vi "FPGA Target_PCIe_7856R.vi"() -> ()   [LabVIEW 2023]
uses:
  <vilib>/Platform/TimedLoop/XDataNode/timing_clust.ctl
  <vilib>/Platform/TimedLoop/XDataNode/nitl_modes.ctl
  <vilib>/Platform/TimedLoop/XDataNode/wakeup.ctl
  <vilib>/rvi/Emulation/niFpgaSctlEmulationGetInTimedLoop.vi
  <vilib>/rvi/Emulation/niFpgaProcessEmulError.vi
  <vilib>/rvi/eio/common/nirviEmuTemplateMethod_errors.vi
  <vilib>/rvi/Emulation/niFpgaGetClockAttributes.vi
  <vilib>/rvi/Emulation/niFpgaEmulationReportErrorSimple.vi
  <vilib>/eio/utilities/niEioResolveVilibRelativePath.vi
  <vilib>/rvi/interface/RandomDataEmulation/niFpgaRandomDataHandleErrors.vi
  <vilib>/rvi/Emulation/niFpgaCriticalErrorInLSC.vi
  Tick Count.vi
  <vilib>/rvi/Memory/Memory_Emulation/nirvimemoryFastEmulation.vi
  <vilib>/rvi/Memory/Memory_Emulation/nirvimemoryEmulation.vi
  <vilib>/rvi/Emulation/niFpgaEmulationIsFPGAContextNoSignature.vi
  <vilib>/rvi/DataTransferAndStorage/Container/Common/niFpgaContainerGetUniqueNameForEmu.vi
  <vilib>/rvi/errors/nirviReportUnexpectedCaseInternalError (U32).vi
  <vilib>/eio/EIONode/EIONode.xnode
  <vilib>/rvi/DataTransferAndStorage/Container/XNode/niFpgaContainer.xnode
  <vilib>/rvi/interface/RandomDataEmulation/nirviRandomDataFpgaReadWriteTemplate.vi
  <vilib>/Platform/TimedLoop/XDataNode/XDataNode.xnode
  <vilib>/rvi/Arithmetic/AddSubMult/XNode/nirviSatArithmetic.xnode
  <vilib>/Platform/TimedLoop/XDataNode/XDNodeRunTimeDep.lvlib
panel:
  out "Move Z Picomotor Direction":bool
  out "Move Z Picomotor":bool
  out "Tick Count(Ticks)":u32
  in  "HoldTimerScale":u64=18446744073709526080
  in  "Feedback1 on  Hold":bool
  out "Feedback2 Error":i32
  out "Feedback1 Error":i32
  out "Feedback2 Boolean":bool
  out "Feedback1 Boolean":bool
  out "ExtraTime 4":fxp<+,64,64>
  in  "DistanceToBulk 3":i16
  in  "DistanceToBulk 2":i16
  out "HasHeldHoldTimeHappend?":bool
  out "Z_axis_-10Vto10V":bool
  out "TraceRetraceFirstUse":bool
  in  "DistanceToBulk":i16
  out "V START":i16
  out "V END":i16
  out "X START":i16
  out "Y START":i16
  out "Z START":i16
  out "X END":i16
  out "Y END":i16
  out "Z END":i16
  out "V2 START":i16
  out "Count Average":i16
  out "AverageSum":i64
  out "IterateHolder":i16
  out "V2 VEl":i16
  out "V2 END":i16
  out "Update Position Loop Wait Time (ms)":u16=1
  out "LineType":i16
  out "V VEl":i16
  out "Z VEL":i16
  out "Y VEL":i16
  out "X VEL":i16
  out "Element":i16
  in  "V on Fly":i16=-32768
  in  "Change V on Fly":bool
  in  "Feedback_Threshold":i64
  in  "FeedBackType":u8
  out "x < y?":bool
  out "ExtraTime 3":fxp<+,64,64>
  in  "P2AvgMinus":i32
  out "ExtraTime 2":fxp<+,64,64>
  in  "P2AvgWhole":i32
  in  "Xoffset":u32
  in  "P":fxp<+/-,32,1>
  in  "Upper limit Of dZ":i32
  in  "FeedBackType 2":u8
  in  "Feedback_Threshold 2":i32
  in  "GreaterThan 2":bool
  in  "GreaterThan":bool
  in  "V2 on Fly":i16=-32768
  in  "Change V on Fly 2":bool
  out "CurrentMeasuredX":i16
  in  "2^(-n)":i16
  out "SampleNum":i16
  in  "Buffer Loop Wait Time (tICKS)":u32=1
  out "SampleIterator":i16
  out "Internal Stop":bool caption="Stop"
  out "MeasuredCurrent":i16=32767
  out "Applied Voltage":i16=-32768
  in  "External Stop":bool caption="Stop"
  in  "External Pause":bool
  out "Applied Z":i16
  out "Applied Y":i16
  out "Applied X":i16
  in  "Internal Pause":bool
  out "Accum Z":i32
  out "Accum I":i32
  out "Accum dV":i32
  out "Accum I2":i32
  out "OnlyStopLineONCE X":bool
  out "Accum Ext ac":i32
  out "Ext amp":i16=32767
  out "Accum Ext phase":i32
  in  "ExpandVelScaller X":i16=-27
  out "LineNumber":u64
  out "WaitingForWayPoints":bool caption="Stop"
  out "HoldTimer (ticks)":u64
  out "MeasuredCurrent 2":i16=32767
  out "Ext Phase":i16=32767
  in  "ExpandVelScaller Y":i16=-27
  in  "ExpandVelScaller Z":i16=-27
  in  "ExpandVelScaller V":i16=-27
  out "Accum I3":i32
  out "MeasuredCurrent 3":i16=32767
  out "MeasuredCurrent 4":i16=32767
  out "Accum Y":i32
  out "Accum X":i32
  out "OnlyStopLineONCE Y":bool
  out "OnlyStopLineONCE Z":bool
  out "OnlyStopLineONCE V":bool
  in  "EndCurrentLine":bool
  out "StopMoveX":bool
  out "StopMoveY":bool
  out "StopMoveZ":bool
  out "StopMoveV":bool
  out "Jump V":bool
  out "Stop Hold Position":bool
  out "Applied Voltage 2":i16
  out "StopMoveV2":bool
  out "Accum dV2":i32
  out "Jump V2":bool
  in  "ExpandVelScaller V2":i16=-27
  out "OnlyStopLineONCE V2":bool
  out "MoveAverage":i16
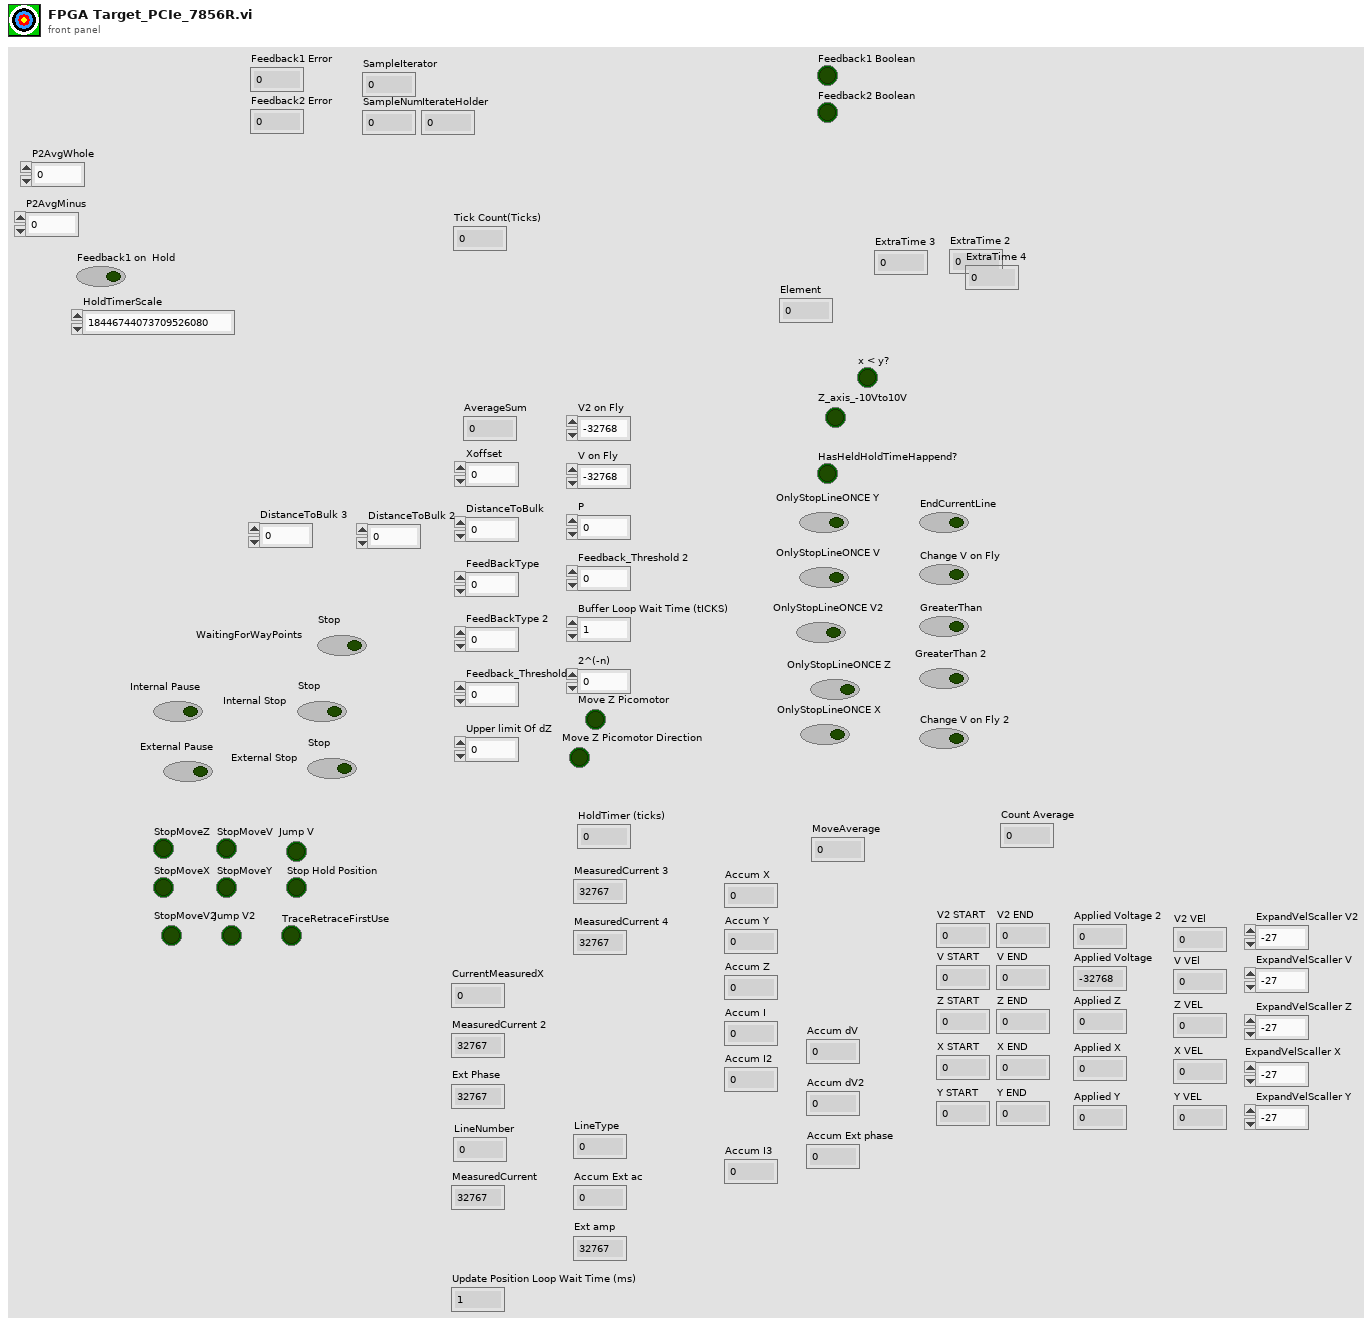
[diagram p1: front panel]
types:
  T1 = typedef "XDNodeRunTimeDep.lvlib/timing_clust.ctl" = cluster{"Expected End [f-1]":u64, "Actual End [f-1]":u64, "Finished Late? [f-1]":bool, "Expected End [i-1]":u64, "Actual End [i-1]":u64, "Finished Late? [i-1]":bool, "Expected Start [i]":u64, "Actual Start [i]":u64, "Expected Start [f]":u64, "Actual Start [f]":u64, "Source Name":string, "Structure Name":string, "Period":i64, "Deadline":i64, "Offset":i64, "Start":i64, "Priority":i32, "Timeout":i32, "Mode":T2, "Wakeup Reason":T3, "Error":errorcluster, "Source Type":string, "Secondary Source Type":string, "Global End Time":u64, "Global Start Time":u64, "Frame Duration":u64, "Iteration Duration":u64, "Assigned CPU":i32, "I/O Scan Engine Mode":u32}
  T2 = typedef "XDNodeRunTimeDep.lvlib/nitl_modes.ctl" = enum32{"No Change", "Process missed periods, maintain original phase", "Discard missed periods, maintain original phase", "Process missed periods, ignore original phase", "Discard missed periods, ignore original phase"}
  T3 = typedef "XDNodeRunTimeDep.lvlib/wakeup.ctl" = enum32{"Normal", "Aborted", "Asynchronous wakeup", "Timing source error", "Timed loop error", "Timeout"}
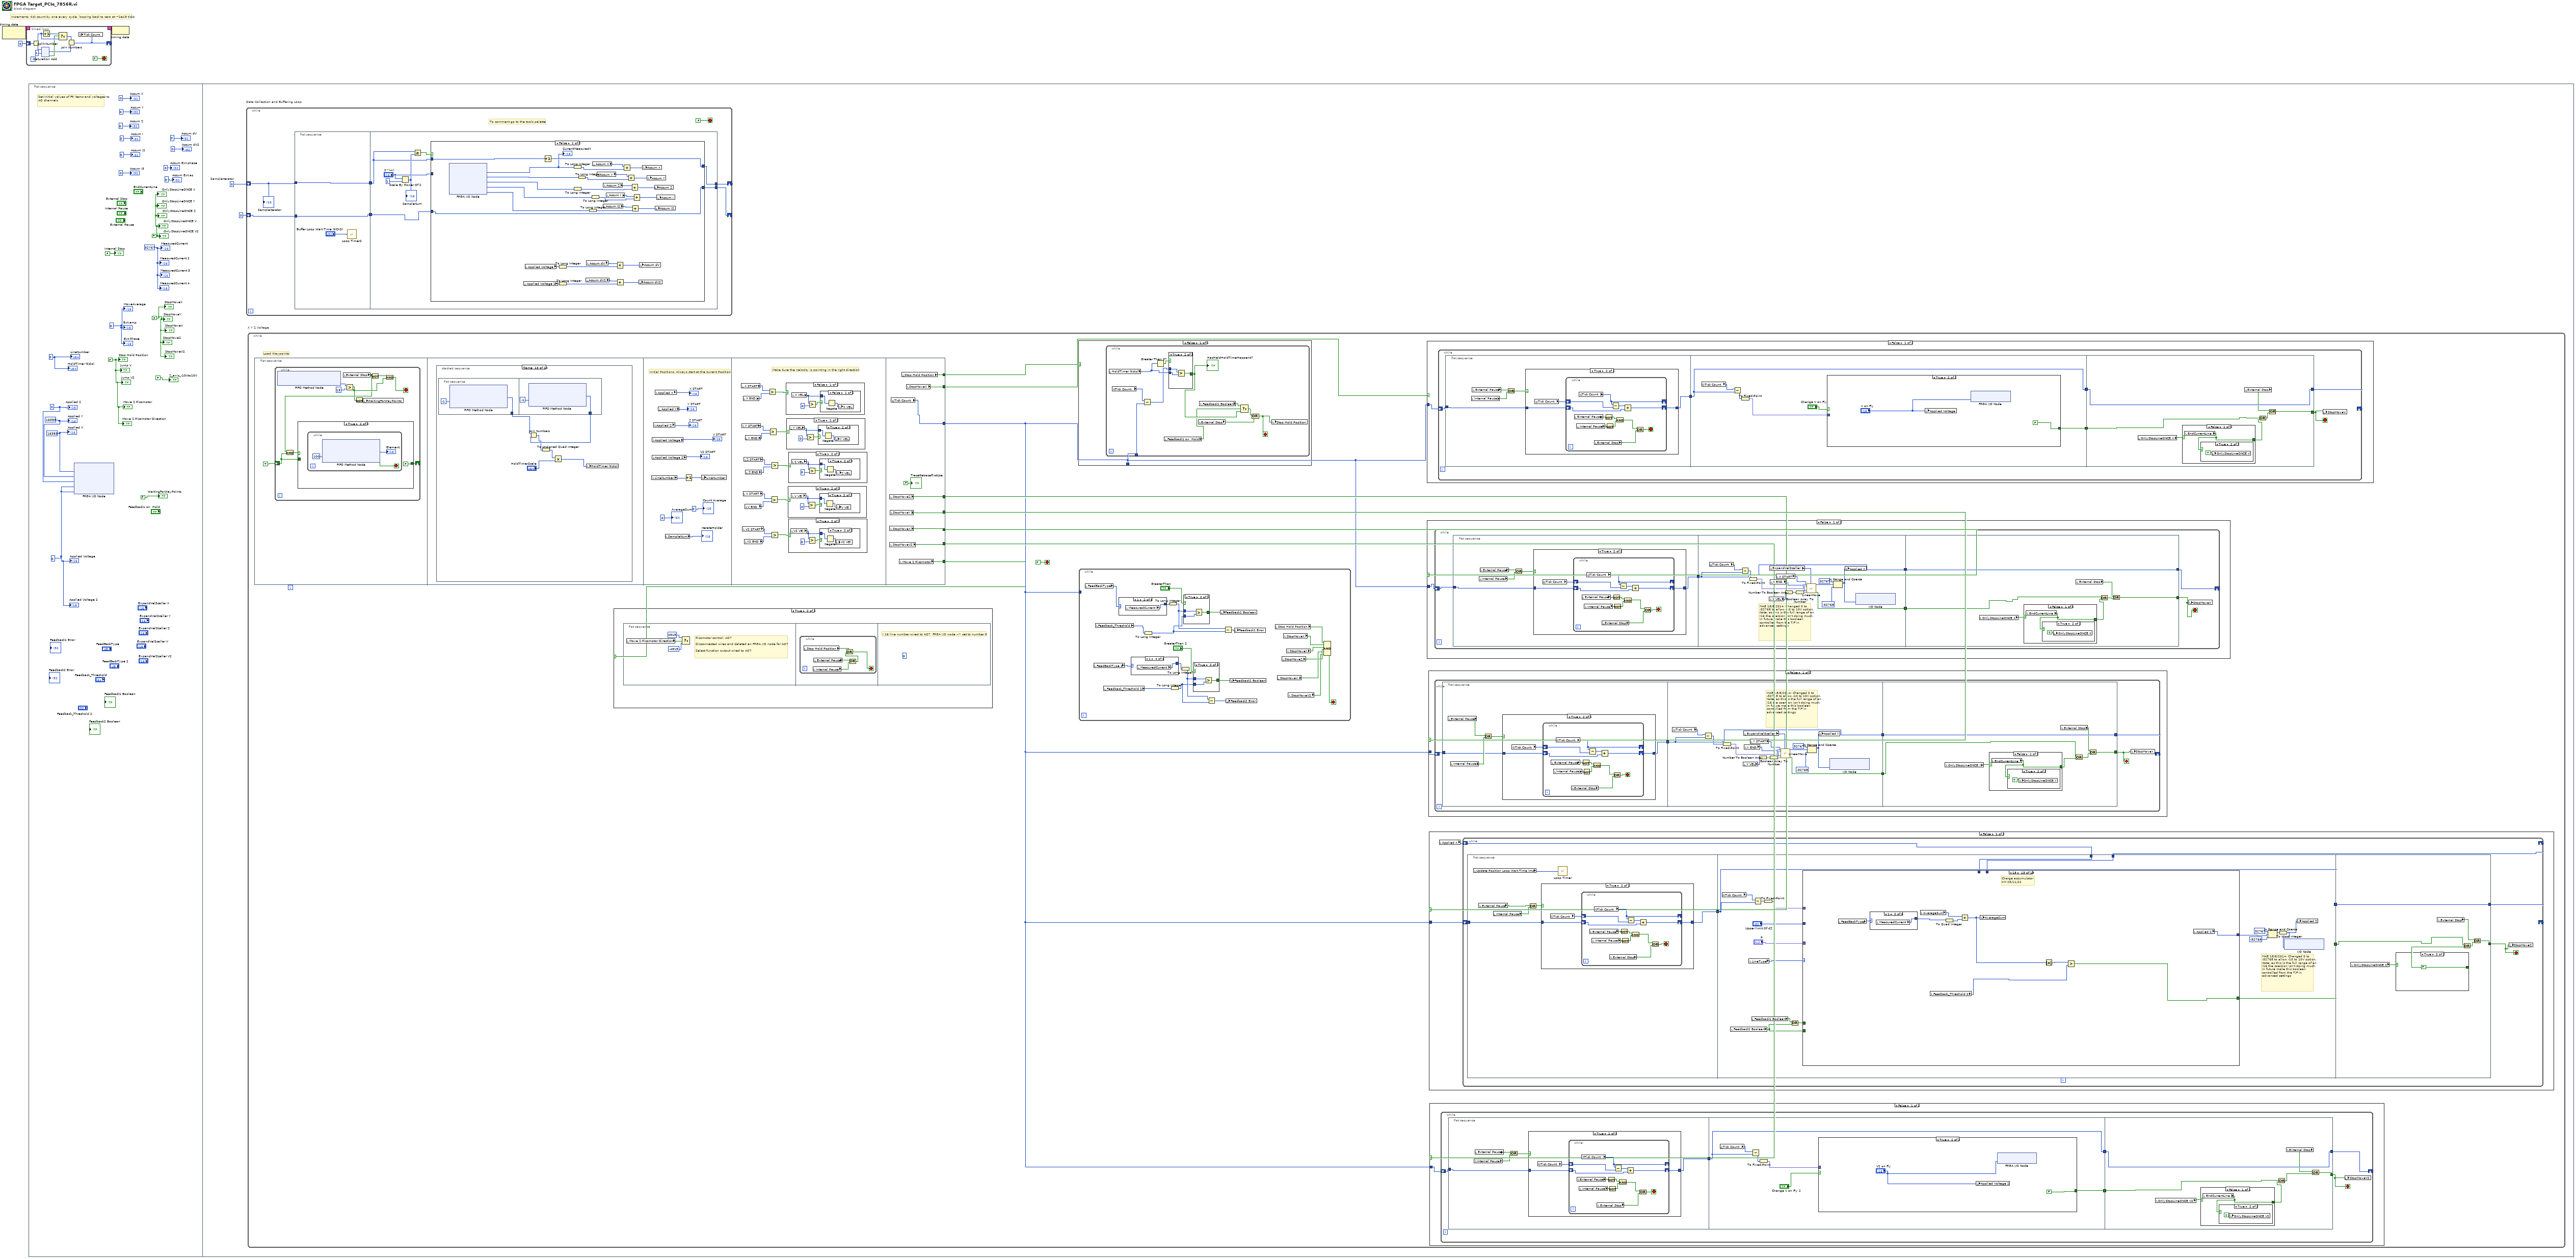
[diagram p0: block diagram]
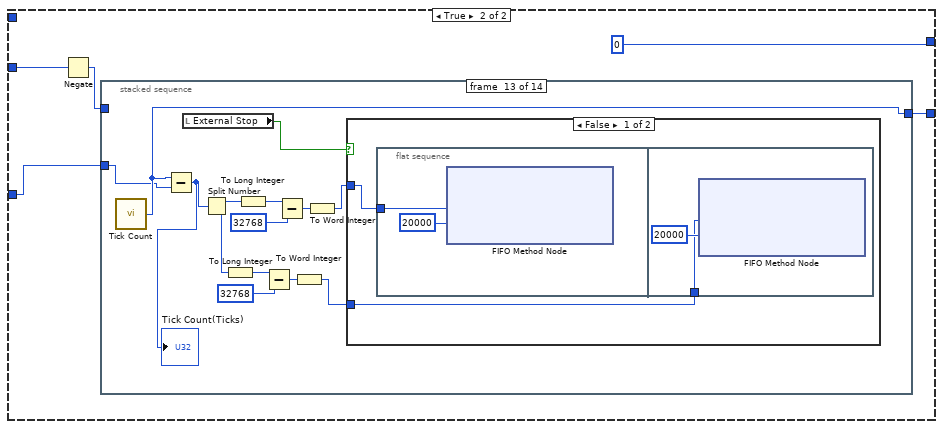
[diagram p2: hidden frame]
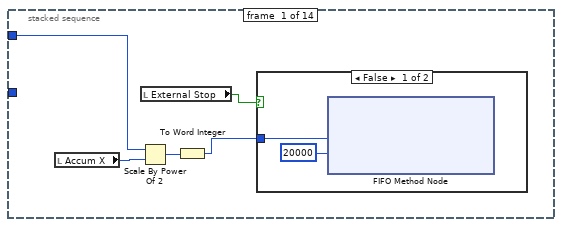
[diagram p3: hidden frame]
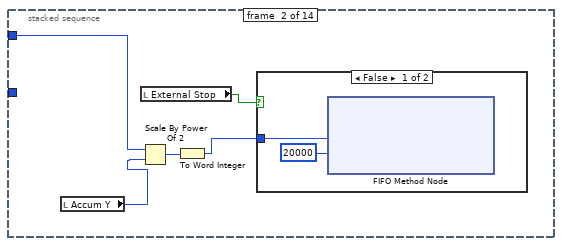
[diagram p5: hidden frame]
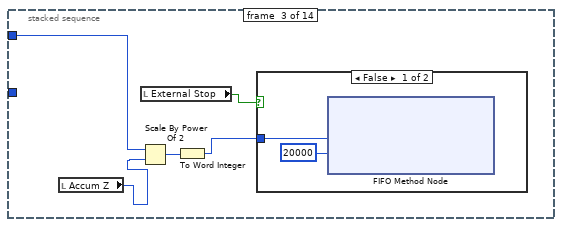
[diagram p7: hidden frame]
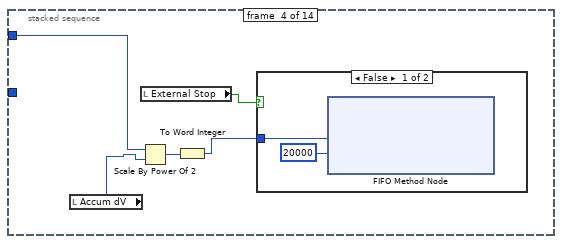
[diagram p9: hidden frame]
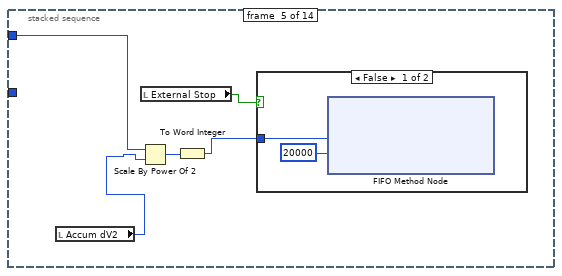
[diagram p11: hidden frame]
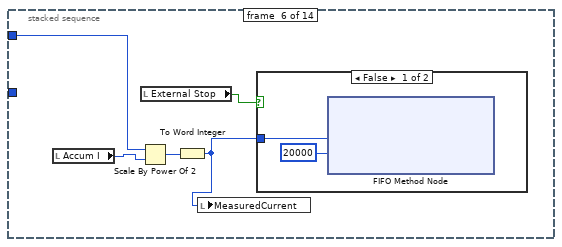
[diagram p13: hidden frame]
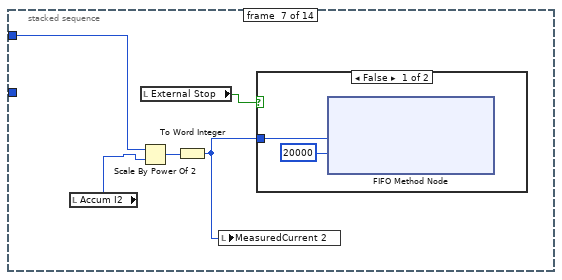
[diagram p15: hidden frame]
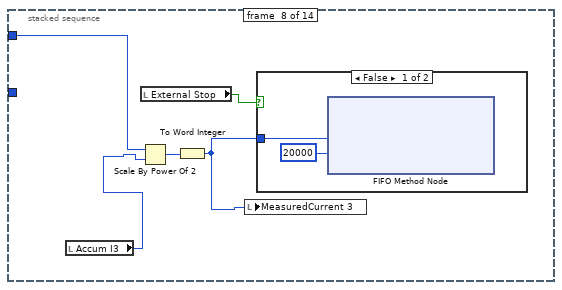
[diagram p17: hidden frame]
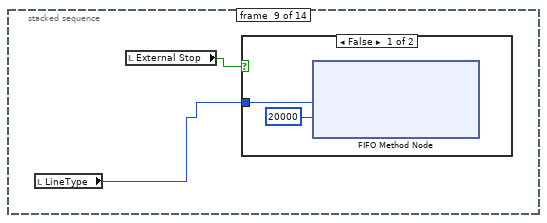
[diagram p19: hidden frame]
diagram:
  # "Increments  tick count by one every cycle, looping back to zero at ~2e19 ticks"
  n1 = node-c288() -> (w3:T1)  [unwired: 1 in]
  n2 = timed-loop {
    timing: w3 -> [_]
    timing-out: [_] -> w2
    shift-right: [w5] -> _
    shift-left: u64 0 -> [w13]
    stop <- FALSE stop-if-true
    n3 = Split Number(x=w13) -> (hi(x)=w10:u32, lo(x)=w12:u32)
    n4 = xnode "Saturation Add"("x"=w12, "y"=u32 1) -> ("x+y"=w6:u32, "overflow"=w7:bool)
    n5 = Increment(x=w10) -> (x+1=w11:u32)
    n6 = Select(t=w11, s=w7, f=w10) -> (s? t:f=w9:u32)
    n7 = Join Numbers(hi=w9, lo=w6) -> ((hi.lo)=w5:u64)
    n8 = global write "Tick Count.vi" "Tick Count"(w5) -> ()
  }
  n9 = flat-sequence {
    frame #0 {
      w28 = i16 0 ("Applied Voltage")
      w33 = FALSE ("OnlyStopLineONCE V2")
      w34 = FALSE ("Internal Stop")
      w29 = FALSE ("Internal Stop")
      w36 = i16 0 ("Applied Volatge")
      w37 = i16 16383 ("Applied Volatge")
      w38 = i16 16383 ("Applied Volatge")
      w32 = u64 0 ("LineNumber")
      w31 = i16 0 ("Ext amp")
      w41 = i16 32767 ("dZ Position")
      # "Set initial values of FP items and voltages to AO channels"
      n10 = xnode "FPGA I/O Node"("Connector0/AO0"=w38, "Connector0/AO1"=w37, "Connector0/AO2"=w36, "Connector0/AO3"=w28, "Connector0/AO4"=w28) -> ()  [unwired: 5 in, 5 out]
      "Internal Stop" <- FALSE ("Internal Stop")
      "MeasuredCurrent" <- w41
      "Applied Voltage" <- w28
      "Applied Z" <- w36
      "Applied Y" <- w37
      "Applied X" <- w38
      "Accum Z" <- 0 ("Applied Volatge")
      "Accum I" <- 0 ("Applied Volatge")
      "Accum dV" <- 0 ("Applied Volatge")
      "Accum I2" <- 0 ("Applied Volatge")
      "OnlyStopLineONCE X" <- w33
      "Accum Ext ac" <- 0 ("Accum Ext ac")
      "Ext amp" <- w31
      "Accum Ext phase" <- 0 ("Accum Ext phase")
      "LineNumber" <- w32
      "WaitingForWayPoints" <- FALSE ("WaitingForWayPoints")
      "HoldTimer (ticks)" <- w32
      "MeasuredCurrent 2" <- w41
      "Ext Phase" <- w31
      "Accum I3" <- 0 ("Applied Volatge")
      "MeasuredCurrent 3" <- w41
      "MeasuredCurrent 4" <- w41
      "Accum Y" <- 0 ("Applied Volatge")
      "Accum X" <- 0 ("Applied Volatge")
      "OnlyStopLineONCE Y" <- w33
      "OnlyStopLineONCE Z" <- w33
      "OnlyStopLineONCE V" <- w33
      "StopMoveX" <- w34
      "StopMoveY" <- w34
      "StopMoveZ" <- w34
      "StopMoveV" <- w34
      "Jump V" <- w29
      "Stop Hold Position" <- w29
      "Applied Voltage 2" <- w28
      "StopMoveV2" <- w34
      "Accum dV2" <- 0 ("Applied Volatge")
      "Jump V2" <- w29
      "OnlyStopLineONCE V2" <- w33
      "MoveAverage" <- w31
      "Z_axis_-10Vto10V" <- FALSE ("Internal Stop")
      "Move Z Picomotor" <- w29
      "Move Z Picomotor Direction" <- w29
    }
    frame #1 {
      w52 = i16 0  # SampleIterator
      n11 = while "Data Collection and Buffering Loop" {
        shift-right: [w57] -> _
        shift-left: w52 -> [w58]
        shift-right: [w55] -> _
        shift-left: u32 0 ("Tick Count(Ticks)") -> [w53]
        stop <- FALSE stop-if-true
        # "To comment go to the tools palette"
        n12 = flat-sequence {
          tunnel: [w62] -> w59
          tunnel: w58 -> [w62]
          tunnel: w53 -> [w60]
          tunnel: [w60] -> w54
          tunnel: w59 -> [w70]
          tunnel: [w69] -> w57
          tunnel: [w64] -> w55
          tunnel: w54 -> [w63]
          frame #0 {
            n13 = call "Loop Timer2"("Count(Ticks)"="Buffer Loop Wait Time (tICKS)") -> ()  [unwired: 1 out]
          }
          frame #1 {
            n14 = Scale By Power Of 2(n="2^(-n)", x=i16 1) -> (x*2^n=w67:i16)
            "SampleNum" <- w67
            n15 = Greater Or Equal?(x=w70, y=w67) -> (x >= y?=w65:bool)
            n16 = case shown="False" w65 {
              tunnel: w70 -> [w101 _]
              tunnel: [w100 i16 0 ("lo")] -> w69
              tunnel: "2^(-n)" -> [_ w105]
              tunnel: [w73 w103] -> w64
              tunnel: w63 -> [w73 w102]
              frame False {
                n17 = xnode "FPGA I/O Node"() -> ("Connector0/AI0"=w78:i16, "Connector0/AI1"=w85:i16, "Connector0/AI2"=w88:i16, "Connector0/AI3"=w72:i16, "Connector0/AI4"=w71:i16)  [unwired: 5 in, 5 out]
                "CurrentMeasuredX" <- w78
                n18 = local read "Applied Voltage 2"() -> (w76:i16)
                n19 = local read "Applied Voltage"() -> (w90:i16)
                n20 = Increment(x=w101) -> (x+1=w100:i16)
                n21 = To Long Integer(number=w90) -> (32bit integer=w89:i32)
                n22 = To Long Integer(number=w76) -> (32bit integer=w77:i32)
                n23 = To Long Integer(number=w88) -> (32bit integer=w86:i32)
                n24 = To Long Integer(number=w78) -> (32bit integer=w79:i32)
                n25 = To Long Integer(number=w85) -> (32bit integer=w84:i32)
                n26 = local read "Accum dV2"() -> (w74:i32)
                n27 = local read "Accum dV"() -> (w92:i32)
                n28 = To Long Integer(number=w71) -> (32bit integer=w94:i32)
                n29 = To Long Integer(number=w72) -> (32bit integer=w97:i32)
                n30 = local read "Accum X"() -> (w80:i32)
                n31 = local read "Accum Y"() -> (w83:i32)
                n32 = local read "Accum I2"() -> (w95:i32)
                n33 = local read "Accum Z"() -> (w87:i32)
                n34 = local read "Accum I"() -> (w98:i32)
                n35 = Add(x=w92, y=w89) -> (x+y=w91:i32)
                n36 = Add(x=w74, y=w77) -> (x+y=w75:i32)
                n37 = Add(x=w80, y=w79) -> (x+y=w81:i32)
                n38 = Add(x=w83, y=w84) -> (x+y=w82:i32)
                n39 = Add(x=w87, y=w86) -> (x+y=w99:i32)
                n40 = Add(x=w95, y=w94) -> (x+y=w93:i32)
                n41 = Add(x=w98, y=w97) -> (x+y=w96:i32)
                n42 = local write "Accum dV2"(w75) -> ()
                n43 = local write "Accum dV"(w91) -> ()
                n44 = local write "Accum X"(w81) -> ()
                n45 = local write "Accum Y"(w82) -> ()
                n46 = local write "Accum Z"(w99) -> ()
                n47 = local write "Accum I2"(w93) -> ()
                n48 = local write "Accum I"(w96) -> ()
              }
              frame True {
                n49 = Negate(x=w105) -> (-x=w104:i16)
                n50 = stacked-sequence {
                  tunnel: w104 -> [w107 w115 w122 w130 w137 w144 w151 w158 _ _ w175 w182 _ _]
                  tunnel: [_ _ _ _ _ _ _ _ _ _ _ _ w188 _] -> w103
                  tunnel: w102 -> [_ _ _ _ _ _ _ _ _ _ _ _ w187 _]
                  frame #0 {
                    n51 = local read "Accum X"() -> (w108:i32)
                    n52 = Scale By Power Of 2(n=w107, x=w108) -> (x*2^n=w109:i32)
                    n53 = local read "External Stop"() -> (w110:bool)
                    n54 = To Word Integer(number=w109) -> (16bit integer=w111:i16)
                    n55 = case shown="False" w110 {
                      tunnel: w111 -> [w112 _]
                      frame False {
                        n56 = xnode ("FIFO Method Node")("Element"=w112, "Timeout"=20000) -> ()  [unwired: 1 in, 2 out]
                      }
                      frame True {
                      }
                    }
                  }
                  frame #1 {
                    n57 = local read "Accum Y"() -> (w114:i32)
                    n58 = Scale By Power Of 2(n=w115, x=w114) -> (x*2^n=w116:i32)
                    n59 = local read "External Stop"() -> (w117:bool)
                    n60 = To Word Integer(number=w116) -> (16bit integer=w118:i16)
                    n61 = case shown="False" w117 {
                      tunnel: w118 -> [w119 _]
                      frame False {
                        n62 = xnode ("FIFO Method Node")("Element"=w119, "Timeout"=20000) -> ()  [unwired: 1 in, 2 out]
                      }
                      frame True {
                      }
                    }
                  }
                  frame #2 {
                    n63 = local read "Accum Z"() -> (w121:i32)
                    n64 = Scale By Power Of 2(n=w122, x=w121) -> (x*2^n=w123:i32)
                    n65 = local read "External Stop"() -> (w124:bool)
                    n66 = To Word Integer(number=w123) -> (16bit integer=w125:i16)
                    n67 = case shown="False" w124 {
                      tunnel: w125 -> [w126 _]
                      frame False {
                        n68 = xnode ("FIFO Method Node")("Element"=w126, "Timeout"=20000) -> ()  [unwired: 1 in, 2 out]
                      }
                      frame True {
                      }
                    }
                  }
                  frame #3 {
                    n69 = local read "Accum dV"() -> (w128:i32)
                    n70 = Scale By Power Of 2(n=w130, x=w128) -> (x*2^n=w131:i32)
                    n71 = local read "External Stop"() -> (w132:bool)
                    n72 = To Word Integer(number=w131) -> (16bit integer=w129:i16)
                    n73 = case shown="False" w132 {
                      tunnel: w129 -> [w133 _]
                      frame False {
                        n74 = xnode ("FIFO Method Node")("Element"=w133, "Timeout"=20000) -> ()  [unwired: 1 in, 2 out]
                      }
                      frame True {
                      }
                    }
                  }
                  frame #4 {
                    n75 = local read "Accum dV2"() -> (w135:i32)
                    n76 = Scale By Power Of 2(n=w137, x=w135) -> (x*2^n=w138:i32)
                    n77 = local read "External Stop"() -> (w139:bool)
                    n78 = To Word Integer(number=w138) -> (16bit integer=w136:i16)
                    n79 = case shown="False" w139 {
                      tunnel: w136 -> [w140 _]
                      frame False {
                        n80 = xnode ("FIFO Method Node")("Element"=w140, "Timeout"=20000) -> ()  [unwired: 1 in, 2 out]
                      }
                      frame True {
                      }
                    }
                  }
                  frame #5 {
                    n81 = local read "Accum I"() -> (w143:i32)
                    n82 = Scale By Power Of 2(n=w144, x=w143) -> (x*2^n=w145:i32)
                    n83 = local read "External Stop"() -> (w146:bool)
                    n84 = To Word Integer(number=w145) -> (16bit integer=w142:i16)
                    n85 = local write "MeasuredCurrent"(w142) -> ()
                    n86 = case shown="False" w146 {
                      tunnel: w142 -> [w147 _]
                      frame False {
                        n87 = xnode ("FIFO Method Node")("Element"=w147, "Timeout"=20000) -> ()  [unwired: 1 in, 2 out]
                      }
                      frame True {
                      }
                    }
                  }
                  frame #6 {
                    n88 = local read "Accum I2"() -> (w150:i32)
                    n89 = Scale By Power Of 2(n=w151, x=w150) -> (x*2^n=w152:i32)
                    n90 = local read "External Stop"() -> (w153:bool)
                    n91 = To Word Integer(number=w152) -> (16bit integer=w149:i16)
                    n92 = local write "MeasuredCurrent 2"(w149) -> ()
                    n93 = case shown="False" w153 {
                      tunnel: w149 -> [w154 _]
                      frame False {
                        n94 = xnode ("FIFO Method Node")("Element"=w154, "Timeout"=20000) -> ()  [unwired: 1 in, 2 out]
                      }
                      frame True {
                      }
                    }
                  }
                  frame #7 {
                    n95 = local read "Accum I3"() -> (w157:i32)
                    n96 = Scale By Power Of 2(n=w158, x=w157) -> (x*2^n=w159:i32)
                    n97 = local read "External Stop"() -> (w160:bool)
                    n98 = To Word Integer(number=w159) -> (16bit integer=w156:i16)
                    n99 = local write "MeasuredCurrent 3"(w156) -> ()
                    n100 = case shown="False" w160 {
                      tunnel: w156 -> [w161 _]
                      frame False {
                        n101 = xnode ("FIFO Method Node")("Element"=w161, "Timeout"=20000) -> ()  [unwired: 1 in, 2 out]
                      }
                      frame True {
                      }
                    }
                  }
                  frame #8 {
                    n102 = local read "LineType"() -> (w163:i16)
                    n103 = local read "External Stop"() -> (w164:bool)
                    n104 = case shown="False" w164 {
                      tunnel: w163 -> [w165 _]
                      frame False {
                        n105 = xnode ("FIFO Method Node")("Element"=w165, "Timeout"=20000) -> ()  [unwired: 1 in, 2 out]
                      }
                      frame True {
                      }
                    }
                  }
                  frame #9 {
                    n106 = local read "LineNumber"() -> (w168:u64)
                    n107 = local read "External Stop"() -> (w169:bool)
                    n108 = To Word Integer(number=w168) -> (16bit integer=w167:i16)
                    n109 = case shown="False" w169 {
                      tunnel: w167 -> [w170 _]
                      frame False {
                        n110 = xnode ("FIFO Method Node")("Element"=w170, "Timeout"=20000) -> ()  [unwired: 1 in, 2 out]
                      }
                      frame True {
                      }
                    }
                  }
                  frame #10 {
                    n111 = local read "Accum Ext ac"() -> (w174:i32)
                    n112 = local read "External Stop"() -> (w176:bool)
                    n113 = Scale By Power Of 2(n=w175, x=w174) -> (x*2^n=w173:i32)
                    n114 = To Word Integer(number=w173) -> (16bit integer=w172:i16)
                    n115 = case shown="False" w176 {
                      tunnel: w172 -> [w177 _]
                      frame False {
                        n116 = xnode ("FIFO Method Node")("Element"=w177, "Timeout"=20000) -> ()  [unwired: 1 in, 2 out]
                      }
                      frame True {
                      }
                    }
                    n117 = local write "Ext amp"(w172) -> ()
                  }
                  frame #11 {
                    n118 = local read "Accum Ext phase"() -> (w180:i32)
                    n119 = local read "External Stop"() -> (w183:bool)
                    n120 = Scale By Power Of 2(n=w182, x=w180) -> (x*2^n=w181:i32)
                    n121 = To Word Integer(number=w181) -> (16bit integer=w179:i16)
                    n122 = local write "Ext Phase"(w179) -> ()
                    n123 = case shown="False" w183 {
                      tunnel: w179 -> [w184 _]
                      frame False {
                        n124 = xnode ("FIFO Method Node")("Element"=w184, "Timeout"=20000) -> ()  [unwired: 1 in, 2 out]
                      }
                      frame True {
                      }
                    }
                  }
                  frame #12 {
                    n125 = call "Tick Count"() -> ("Tick Count(Ticks)"=w188:u32)
                    n126 = Subtract(x=w188, y=w187) -> (x-y=w186:u32)
                    "Tick Count(Ticks)" <- w186
                    n127 = local read "External Stop"() -> (w199:bool)
                    n128 = Split Number(x=w186) -> (hi(x)=w198:u16, lo(x)=w190:u16)
                    n129 = To Long Integer(number=w190) -> (32bit integer=w191:i32)
                    n130 = To Long Integer(number=w198) -> (32bit integer=w197:i32)
                    n131 = Subtract(x=w191, y=32768) -> (x-y=w193:i32)
                    n132 = Subtract(x=w197, y=32768) -> (x-y=w195:i32)
                    n133 = To Word Integer(number=w193) -> (16bit integer=w189:i16)
                    n134 = To Word Integer(number=w195) -> (16bit integer=w194:i16)
                    n135 = case shown="False" w199 {
                      tunnel: w194 -> [w201 _]
                      tunnel: w189 -> [w200 _]
                      frame False {
                        n136 = flat-sequence {
                          tunnel: w201 -> [w202]
                          tunnel: w200 -> [w204]
                          frame #0 {
                            n137 = xnode ("FIFO Method Node")("Element"=w202, "Timeout"=20000) -> ()  [unwired: 1 in, 2 out]
                          }
                          frame #1 {
                            n138 = xnode ("FIFO Method Node")("Element"=w204, "Timeout"=20000) -> ()  [unwired: 1 in, 2 out]
                          }
                        }
                      }
                      frame True {
                      }
                    }
                  }
                  frame #13 {
                    n139 = local write "Accum dV"(0 ("MeasuredCurrent")) -> ()
                    n140 = local write "Accum Z"(0 ("MeasuredCurrent")) -> ()
                    n141 = local write "Accum dV2"(0 ("Accum Ext ac")) -> ()
                    n142 = local write "Accum I2"(0 ("MeasuredCurrent")) -> ()
                    n143 = local write "Accum I"(0 ("MeasuredCurrent")) -> ()
                    n144 = local write "Accum Y"(0 ("Accum Ext ac")) -> ()
                    n145 = local write "Accum X"(0 ("MeasuredCurrent")) -> ()
                    n146 = local write "Accum Ext ac"(0 ("Accum Ext ac")) -> ()
                    n147 = local write "Accum I3"(0 ("Accum Ext ac")) -> ()
                    n148 = local write "Accum Ext phase"(0 ("Accum Ext phase")) -> ()
                  }
                }
              }
            }
          }
        }
        "SampleIterator" <- w58
      }
      n149 = while "X Y Z Voltage" {
        stop <- FALSE stop-if-true
        # "Load Waypoints"
        n150 = flat-sequence {
          tunnel: [w1142] -> w217
          tunnel: [w1141] -> w223
          tunnel: [w1140] -> w222
          tunnel: [w1139] -> w221
          tunnel: [w1138] -> w220
          tunnel: [w1137] -> w219
          tunnel: [w1135] -> w218
          tunnel: [w1134] -> w216
          frame #0 {
            n151 = while {
              shift-right: [w938] -> _
              shift-left: TRUE ("WaitingForWayPoints") -> [w939]
              stop <- w942 stop-if-true
              n152 = xnode ("FIFO Method Node")() -> ("Number of Elements to Read"=w947:u32)  [unwired: 1 in, 1 out]
              n153 = local read "External Stop"() -> (w940:bool)
              n154 = And(x=w940, y=w939) -> (x .and. y?=w941:bool)
              n155 = case shown="True" w941 {
                tunnel: w939 -> [w948 _]
                tunnel: [w948 FALSE ("WaitingForWayPoints")] -> w938
                frame False {
                }
                frame True {
                  n156 = while {
                    stop <- w950 stop-if-true
                    n157 = xnode ("FIFO Method Node")("Timeout"=100) -> ("Element"=→"Element":i16, "Timed Out?"=w950:bool)  [unwired: 1 in, 1 out]
                  }
                }
              }
              n158 = Greater?(x=w947, y=u32 13) -> (0:w943:bool)
              n159 = Not(x=w943) -> (.not. x?=w945:bool)
              n160 = local write "WaitingForWayPoints"(w945) -> ()
              n161 = Not(x=w940) -> (.not. x?=w944:bool)
              n162 = And(x=w944, y=w943) -> (x .and. y?=w942:bool)
            }
          }
          frame #1 {
            n163 = stacked-sequence {
              frame #0 {
                n164 = xnode ("FIFO Method Node")("Timeout"=-1) -> ("Element"=→"LineType":i16)  [unwired: 1 in, 2 out]
              }
              frame #1 {
                n165 = xnode ("FIFO Method Node")("Timeout"=-1) -> ("Element"=→"X VEL":i16)  [unwired: 1 in, 2 out]
              }
              frame #2 {
                n166 = xnode ("FIFO Method Node")("Timeout"=-1) -> ("Element"=→"Y VEL":i16)  [unwired: 1 in, 2 out]
              }
              frame #3 {
                n167 = xnode ("FIFO Method Node")("Timeout"=-1) -> ("Element"=→"Z VEL":i16)  [unwired: 1 in, 2 out]
              }
              frame #4 {
                n168 = xnode ("FIFO Method Node")("Timeout"=-1) -> ("Element"=→"V VEl":i16)  [unwired: 1 in, 2 out]
              }
              frame #5 {
                n169 = xnode ("FIFO Method Node")("Timeout"=-1) -> ("Element"=→"V2 VEl":i16)  [unwired: 1 in, 2 out]
              }
              frame #6 {
                n170 = xnode ("FIFO Method Node")("Timeout"=-1) -> ("Element"=→"X END":i16)  [unwired: 1 in, 2 out]
              }
              frame #7 {
                n171 = xnode ("FIFO Method Node")("Timeout"=-1) -> ("Element"=→"Y END":i16)  [unwired: 1 in, 2 out]
              }
              frame #8 {
                n172 = xnode ("FIFO Method Node")("Timeout"=-1) -> ("Element"=w970:i16)  [unwired: 1 in, 2 out]
                n173 = local read "LineType"() -> (w971:i16)
                n174 = case shown="13" w971 {
                  tunnel: [w973 w978 w990 w1002 w1010] -> w969
                  tunnel: w970 -> [w973 _ _ _ _]
                  frame 0..2, Default {
                    # "Normal Move"
                  }
                  frame 3 {
                    # "Bulk At End Of line - Retract"
                    n175 = local read "Z_axis_-10Vto10V"() -> (w977:bool)
                    n176 = local read "Applied Z"() -> (w985:i16)
                    n177 = Select(t=-32768 ("lower limit"), s=w977, f=0 ("lower limit")) -> (s? t:f=w976:i32)
                    n178 = To Long Integer(number=w985) -> (32bit integer=w982:i32)
                    n179 = To Long Integer(number="DistanceToBulk") -> (32bit integer=w983:i32)
                    n180 = Add(x=w982, y=w983) -> (x+y=w981:i32)
                    n181 = In Range and Coerce(upper limit=32767, x=w981, lower limit=w976) -> (coerced(x)=w979:i32)  [unwired: 1 out]
                    n182 = To Word Integer(number=w979) -> (16bit integer=w978:i16)
                  }
                  frame 12 {
                    # "Bulk At End Of line - Retract"
                    n183 = local read "Z_axis_-10Vto10V"() -> (w989:bool)
                    n184 = local read "Applied Z"() -> (w997:i16)
                    n185 = Select(t=-32768 ("lower limit"), s=w989, f=0 ("lower limit")) -> (s? t:f=w988:i32)
                    n186 = To Long Integer(number=w997) -> (32bit integer=w994:i32)
                    n187 = To Long Integer(number="DistanceToBulk 2") -> (32bit integer=w995:i32)
                    n188 = Add(x=w994, y=w995) -> (x+y=w993:i32)
                    n189 = In Range and Coerce(upper limit=32767, x=w993, lower limit=w988) -> (coerced(x)=w991:i32)  [unwired: 1 out]
                    n190 = To Word Integer(number=w991) -> (16bit integer=w990:i16)
                  }
                  frame 13 {
                    # "Bulk At End Of line - Retract"
                    n191 = local read "Z_axis_-10Vto10V"() -> (w1001:bool)
                    n192 = local read "Applied Z"() -> (w1009:i16)
                    n193 = Select(t=-32768 ("lower limit"), s=w1001, f=0 ("lower limit")) -> (s? t:f=w1000:i32)
                    n194 = To Long Integer(number=w1009) -> (32bit integer=w1006:i32)
                    n195 = To Long Integer(number="DistanceToBulk 3") -> (32bit integer=w1007:i32)
                    n196 = Add(x=w1006, y=w1007) -> (x+y=w1005:i32)
                    n197 = In Range and Coerce(upper limit=32767, x=w1005, lower limit=w1000) -> (coerced(x)=w1003:i32)  [unwired: 1 out]
                    n198 = To Word Integer(number=w1003) -> (16bit integer=w1002:i16)
                  }
                  frame 4..7 {
                    # "Start at current hieght"
                    n199 = local read "Applied Z"() -> (w1010:i16)
                  }
                }
                "Z END" <- w969
              }
              frame #9 {
                n200 = xnode ("FIFO Method Node")("Timeout"=-1) -> ("Element"=→"V END":i16)  [unwired: 1 in, 2 out]
              }
              frame #10 {
                n201 = xnode ("FIFO Method Node")("Timeout"=-1) -> ("Element"=→"V2 END":i16)  [unwired: 1 in, 2 out]
              }
              frame #11 {
                n202 = xnode ("FIFO Method Node")("Timeout"=-1) -> ("Element"=w1016:i16)  [unwired: 1 in, 2 out]
                n203 = To Unsigned Word Integer(number=w1016) -> (unsigned 16bit integer=→"Update Position Loop Wait Time (ms)":u16)
              }
              frame #12 {
                n204 = flat-sequence {
                  tunnel: [w1024] -> w1020
                  tunnel: [w1026] -> w1019
                  frame #0 {
                    n205 = xnode ("FIFO Method Node")("Timeout"=-1) -> ("Element"=w1024:i16)  [unwired: 1 in, 2 out]
                  }
                  frame #1 {
                    n206 = xnode ("FIFO Method Node")("Timeout"=-1) -> ("Element"=w1026:i16)  [unwired: 1 in, 2 out]
                  }
                }
                n207 = Join Numbers(hi=w1020, lo=w1019) -> ((hi.lo)=w1018:u32)
                n208 = To Unsigned Quad Integer(1:w1018) -> (0:w1023:u64)
                n209 = Multiply(x=w1023, y="HoldTimerScale") -> (x*y=w1021:u64)
                n210 = local write "HoldTimer (ticks)"(w1021) -> ()
              }
              frame #13 {
                n211 = xnode ("FIFO Method Node")("Timeout"=-1) -> ("Element"=w1037:i16)  [unwired: 1 in, 2 out]
                n212 = Number To Boolean Array(number=w1037) -> (Boolean array=w1028:bool[])
                n213 = Index Array(array=w1028, index=0) -> (element=w1042:bool)
                n214 = Index Array(array=w1028, index=1) -> (element=w1043:bool)
                n215 = Index Array(array=w1028, index=2) -> (element=w1047:bool)
                n216 = Index Array(array=w1028, index=4) -> (element=w1052:bool)
                n217 = Index Array(array=w1028, index=5) -> (element=w1036:bool)
                n218 = Index Array(array=w1028, index=3) -> (element=w1044:bool)
                n219 = Index Array(array=w1028, index=10) -> (element=w1030:bool)
                n220 = Index Array(array=w1028, index=9) -> (element=w1031:bool)
                n221 = Index Array(array=w1028, index=6) -> (element=w1054:bool)
                n222 = Not(x=w1044) -> (.not. x?=w1051:bool)
                n223 = Not(x=w1042) -> (.not. x?=w1048:bool)
                n224 = Not(x=w1036) -> (.not. x?=w1035:bool)
                n225 = Index Array(array=w1028, index=7) -> (element=w1057:bool)
                n226 = Index Array(array=w1028, index=8) -> (element=w1033:bool)
                n227 = Not(x=w1047) -> (.not. x?=w1050:bool)
                n228 = Not(x=w1043) -> (.not. x?=w1049:bool)
                n229 = local write "StopMoveX"(w1048) -> ()
                n230 = local write "Stop Hold Position"(w1035) -> ()
                n231 = Not(x=w1054) -> (.not. x?=w1055:bool)
                n232 = local write "Move Z Picomotor Direction"(w1030) -> ()
                n233 = local write "StopMoveY"(w1049) -> ()
                n234 = local write "StopMoveZ"(w1050) -> ()
                n235 = local write "StopMoveV2"(w1055) -> ()
                n236 = local write "StopMoveV"(w1051) -> ()
                n237 = local write "Move Z Picomotor"(w1031) -> ()
                n238 = local write "Jump V"(w1052) -> ()
                n239 = local write "Feedback1 on  Hold"(w1033) -> ()
                n240 = local write "Jump V2"(w1057) -> ()
              }
            }
          }
          frame #2 {
            # "Initial Positions, Always start at the current Position"
            n241 = local read "LineNumber"() -> (w1064:u64)
            n242 = local read "Applied Voltage"() -> (→"V START":i16)
            n243 = local read "Applied Voltage 2"() -> (→"V2 START":i16)
            n244 = local read "Applied Z"() -> (→"Z START":i16)
            n245 = local read "Applied X"() -> (→"X START":i16)
            n246 = local read "Applied Y"() -> (→"Y START":i16)
            n247 = local read "SampleNum"() -> (→"IterateHolder":i16)
            n248 = Increment(x=w1064) -> (x+1=w1063:u64)
            n249 = local write "LineNumber"(w1063) -> ()
            "Count Average" <- i16 0
            "AverageSum" <- i64 0 ("LineNumber")
          }
          frame #3 {
            # "Make Sure the Velocity is pointing in the right direction"
            n250 = local read "X START"() -> (w1083:i16)
            n251 = local read "Y START"() -> (w1078:i16)
            n252 = local read "V2 START"() -> (w1071:i16)
            n253 = local read "X END"() -> (w1082:i16)
            n254 = local read "V START"() -> (w1072:i16)
            n255 = local read "Z START"() -> (w1077:i16)
            n256 = local read "V2 END"() -> (w1070:i16)
            n257 = local read "V END"() -> (w1073:i16)
            n258 = local read "Y END"() -> (w1079:i16)
            n259 = local read "Z END"() -> (w1076:i16)
            n260 = Greater?(x=w1083, y=w1082) -> (0:w1081:bool)
            n261 = Greater?(x=w1078, y=w1079) -> (0:w1080:bool)
            n262 = Greater?(x=w1072, y=w1073) -> (0:w1074:bool)
            n263 = Greater?(x=w1077, y=w1076) -> (0:w1075:bool)
            n264 = Greater?(x=w1071, y=w1070) -> (0:w1069:bool)
            n265 = case shown="False" w1081 {
              frame False {
                n266 = local read "X VEL"() -> (w1124:i16)
                n267 = Greater?(x=w1124, y=i16 0) -> (0:w1125:bool)
                n268 = case shown="False" w1125 {
                  tunnel: w1124 -> [w1128 _]
                  frame False {
                    n269 = Negate(x=w1128) -> (-x=w1127:i16)
                    n270 = local write "X VEL"(w1127) -> ()
                  }
                  frame True {
                  }
                }
              }
              frame True {
                n271 = local read "X VEL"() -> (w1129:i16)
                n272 = Greater?(x=w1129, y=i16 0) -> (0:w1130:bool)
                n273 = case shown="True" w1130 {
                  tunnel: w1129 -> [_ w1133]
                  frame False {
                  }
                  frame True {
                    n274 = Negate(x=w1133) -> (-x=w1132:i16)
                    n275 = local write "X VEL"(w1132) -> ()
                  }
                }
              }
            }
            n276 = case shown="True" w1080 {
              frame False {
                n277 = local read "Y VEL"() -> (w1114:i16)
                n278 = Greater?(x=w1114, y=i16 0) -> (0:w1115:bool)
                n279 = case shown="False" w1115 {
                  tunnel: w1114 -> [w1118 _]
                  frame False {
                    n280 = Negate(x=w1118) -> (-x=w1117:i16)
                    n281 = local write "Y VEL"(w1117) -> ()
                  }
                  frame True {
                  }
                }
              }
              frame True {
                n282 = local read "Y VEL"() -> (w1119:i16)
                n283 = Greater?(x=w1119, y=i16 0) -> (0:w1120:bool)
                n284 = case shown="True" w1120 {
                  tunnel: w1119 -> [_ w1123]
                  frame False {
                  }
                  frame True {
                    n285 = Negate(x=w1123) -> (-x=w1122:i16)
                    n286 = local write "Y VEL"(w1122) -> ()
                  }
                }
              }
            }
            n287 = case shown="True" w1074 {
              frame False {
                n288 = local read "V VEl"() -> (w1094:i16)
                n289 = Greater?(x=w1094, y=i16 0) -> (0:w1095:bool)
                n290 = case shown="False" w1095 {
                  tunnel: w1094 -> [w1098 _]
                  frame False {
                    n291 = Negate(x=w1098) -> (-x=w1097:i16)
                    n292 = local write "V VEl"(w1097) -> ()
                  }
                  frame True {
                  }
                }
              }
              frame True {
                n293 = local read "V VEl"() -> (w1099:i16)
                n294 = Greater?(x=w1099, y=i16 0) -> (0:w1100:bool)
                n295 = case shown="True" w1100 {
                  tunnel: w1099 -> [_ w1103]
                  frame False {
                  }
                  frame True {
                    n296 = Negate(x=w1103) -> (-x=w1102:i16)
                    n297 = local write "V VEl"(w1102) -> ()
                  }
                }
              }
            }
            n298 = case shown="True" w1075 {
              frame False {
                n299 = local read "Z VEL"() -> (w1104:i16)
                n300 = Greater?(x=w1104, y=i16 0) -> (0:w1105:bool)
                n301 = case shown="False" w1105 {
                  tunnel: w1104 -> [w1108 _]
                  frame False {
                    n302 = Negate(x=w1108) -> (-x=w1107:i16)
                    n303 = local write "Z VEL"(w1107) -> ()
                  }
                  frame True {
                  }
                }
              }
              frame True {
                n304 = local read "Z VEL"() -> (w1109:i16)
                n305 = Greater?(x=w1109, y=i16 0) -> (0:w1110:bool)
                n306 = case shown="True" w1110 {
                  tunnel: w1109 -> [_ w1113]
                  frame False {
                  }
                  frame True {
                    n307 = Negate(x=w1113) -> (-x=w1112:i16)
                    n308 = local write "Z VEL"(w1112) -> ()
                  }
                }
              }
            }
            n309 = case shown="True" w1069 {
              frame False {
                n310 = local read "V2 VEl"() -> (w1084:i16)
                n311 = Greater?(x=w1084, y=i16 0) -> (0:w1085:bool)
                n312 = case shown="False" w1085 {
                  tunnel: w1084 -> [w1088 _]
                  frame False {
                    n313 = Negate(x=w1088) -> (-x=w1087:i16)
                    n314 = local write "V2 VEl"(w1087) -> ()
                  }
                  frame True {
                  }
                }
              }
              frame True {
                n315 = local read "V2 VEl"() -> (w1089:i16)
                n316 = Greater?(x=w1089, y=i16 0) -> (0:w1090:bool)
                n317 = case shown="True" w1090 {
                  tunnel: w1089 -> [_ w1093]
                  frame False {
                  }
                  frame True {
                    n318 = Negate(x=w1093) -> (-x=w1092:i16)
                    n319 = local write "V2 VEl"(w1092) -> ()
                  }
                }
              }
            }
          }
          frame #4 {
            n320 = local read "StopMoveZ"() -> (w1138:bool)
            n321 = local read "StopMoveX"() -> (w1140:bool)
            n322 = local read "StopMoveV2"() -> (w1137:bool)
            n323 = local read "StopMoveY"() -> (w1139:bool)
            n324 = global read "Tick Count.vi" "Tick Count"() -> (w1142:u64)
            n325 = local read "Move Z Picomotor"() -> (w1134:bool)
            n326 = local read "Stop Hold Position"() -> (w1135:bool)
            n327 = local read "StopMoveV"() -> (w1141:bool)
            "TraceRetraceFirstUse" <- FALSE ("Boolean")
          }
        }
        n328 = case shown="True" w216 {
          frame False {
          }
          frame True {
            n329 = flat-sequence {
              frame #0 {
                # "Picomotor control: AO7\n\nDisconnected wires and deleted an FPGA I/O node for AO7\n\nSelect function output wired to AO7"
                n330 = local read "Move Z Picomotor Direction"() -> (w225:bool)
                n331 = Select(t=i16 4915 ("LineNumber"), s=w225, f=i16 -4915 ("LineNumber")) -> ()  [unwired: 1 out]
              }
              frame #1 {
                n332 = while {
                  stop <- w228 stop-if-true
                  n333 = local read "Stop Hold Position"() -> (w232:bool)
                  n334 = local read "Internal Pause"() -> (w231:bool)
                  n335 = local read "External Pause"() -> (w230:bool)
                  n336 = Or(x=w230, y=w231) -> (x .or. y?=w229:bool)
                  n337 = Or(x=w232, y=w229) -> (x .or. y?=w228:bool)
                }
              }
              frame #2 {
                (unwired) i16 0 ("LineNumber")
                # "I 16 line number wired to AO7  FPGA I/O node --> set to number 0"
              }
            }
          }
        }
        n338 = case shown="False" w218 {
          tunnel: w217 -> [w280 _]
          frame False {
            n339 = while {
              tunnel: w280 -> [w288]
              stop <- w284 stop-if-true
              n340 = local read "HoldTimer (ticks)"() -> (w290:u64)
              n341 = global read "Tick Count.vi" "Tick Count"() -> (w289:u64)
              n342 = Subtract(x=w289, y=w288) -> (x-y=w287:u64)
              n343 = Greater Than 0?(x=w290) -> (x > 0?=w291:bool)
              n344 = local read "Feedback1 on  Hold"() -> (w281:bool)
              n345 = case shown="True" w291 {
                tunnel: [FALSE w295] -> w282
                tunnel: w290 -> [_ w294]
                tunnel: w287 -> [_ w293]
                frame False {
                }
                frame True {
                  n346 = Greater?(x=w293, y=w294) -> (0:w295:bool)
                }
              }
              "HasHeldHoldTimeHappend?" <- w282
              n347 = local read "External Stop"() -> (w285:bool)
              n348 = local read "Feedback1 Boolean"() -> (w286:bool)
              n349 = Select(t=w286, s=w281, f=w282) -> (s? t:f=w283:bool)
              n350 = Compound Arithmetic op=OR(w283, w285) -> (w284:bool)
              n351 = local write "Stop Hold Position"(w284) -> ()
            }
          }
          frame True {
          }
        }
        n352 = while {
          tunnel: w217 -> [_]
          stop <- w242 stop-if-true
          n353 = local read "FeedBackType"() -> (w254:u8)
          n354 = local read "FeedBackType 2"() -> (w252:u8)
          n355 = local read "Feedback_Threshold"() -> (w236:i64)
          n356 = local read "Feedback_Threshold 2"() -> (w234:i32)
          n357 = case shown="1" w254 {
            tunnel: [w274 w275 w276 w277 w278 w279] -> w255
            frame 0, Default {
              n358 = local read "Ext amp"() -> (w274:i16)
            }
            frame 1 {
              n359 = local read "MeasuredCurrent"() -> (w275:i16)
            }
            frame 2 {
              n360 = local read "MeasuredCurrent 2"() -> (w276:i16)
            }
            frame 3 {
              n361 = local read "Ext Phase"() -> (w277:i16)
            }
            frame 4 {
              n362 = local read "MeasuredCurrent"() -> (w278:i16)
            }
            frame 5 {
              n363 = local read "MeasuredCurrent 2"() -> (w279:i16)
            }
          }
          n364 = case shown="1" w252 {
            tunnel: [w262 w263 w264 w265 w266 w267] -> w250
            frame 0, Default {
              n365 = local read "Ext amp"() -> (w262:i16)
            }
            frame 4 {
              n366 = local read "MeasuredCurrent 3"() -> (w263:i16)
            }
            frame 5 {
              n367 = local read "MeasuredCurrent 4"() -> (w264:i16)
            }
            frame 1 {
              n368 = local read "MeasuredCurrent"() -> (w265:i16)
            }
            frame 2 {
              n369 = local read "MeasuredCurrent 2"() -> (w266:i16)
            }
            frame 3 {
              n370 = local read "Ext Phase"() -> (w267:i16)
            }
          }
          n371 = To Long Integer(number=w236) -> (32bit integer=w235:i32)
          n372 = To Long Integer(number=w255) -> (32bit integer=w240:i32)
          n373 = To Long Integer(number=w234) -> (32bit integer=w233:i32)
          n374 = To Long Integer(number=w250) -> (32bit integer=w238:i32)
          n375 = case shown="True" "GreaterThan" {
            tunnel: w240 -> [w270 w273]
            tunnel: w235 -> [w269 w271]
            tunnel: [w268 w272] -> w249
            frame False {
              n376 = Less?(x=w270, y=w269) -> (x < y?=w268:bool)
            }
            frame True {
              n377 = Greater?(x=w273, y=w271) -> (0:w272:bool)
            }
          }
          n378 = case shown="True" "GreaterThan 2" {
            tunnel: w238 -> [w258 w261]
            tunnel: w233 -> [w257 w259]
            tunnel: [w256 w260] -> w248
            frame False {
              n379 = Less?(x=w258, y=w257) -> (x < y?=w256:bool)
            }
            frame True {
              n380 = Greater?(x=w261, y=w259) -> (0:w260:bool)
            }
          }
          n381 = Subtract(x=w238, y=w233) -> (x-y=w237:i32)
          n382 = local write "Feedback1 Boolean"(w249) -> ()
          n383 = Subtract(x=w240, y=w235) -> (x-y=w239:i32)
          n384 = local write "Feedback2 Error"(w237) -> ()
          n385 = local write "Feedback2 Boolean"(w248) -> ()
          n386 = local write "Feedback1 Error"(w239) -> ()
          n387 = local read "Stop Hold Position"() -> (w241:bool)
          n388 = local read "StopMoveV"() -> (w244:bool)
          n389 = local read "StopMoveZ"() -> (w245:bool)
          n390 = local read "StopMoveX"() -> (w247:bool)
          n391 = local read "StopMoveY"() -> (w246:bool)
          n392 = local read "StopMoveV2"() -> (w243:bool)
          n393 = Compound Arithmetic op=AND(w241, w247, w246, w245, w244, w243) -> (w242:bool)
        }
        n394 = case shown="False" w223 {
          tunnel: w217 -> [w875 _]
          frame False {
            n395 = while {
              shift-right: [w877] -> _
              shift-left: w875 -> [w880]
              stop <- w876 stop-if-true
              n396 = flat-sequence {
                tunnel: w880 -> [w882]
                tunnel: [w883] -> w881
                tunnel: w881 -> [w908]
                tunnel: [w908] -> w879
                tunnel: [w904] -> w878
                tunnel: [w933] -> w877
                tunnel: w879 -> [w933]
                tunnel: w878 -> [w927]
                tunnel: [w928] -> w876
                frame #0 {
                  n397 = local read "Internal Pause"() -> (w885:bool)
                  n398 = local read "External Pause"() -> (w886:bool)
                  n399 = Or(x=w886, y=w885) -> (x .or. y?=w884:bool)
                  n400 = case shown="True" w884 {
                    tunnel: w882 -> [w887 w890]
                    tunnel: [w887 w888] -> w883
                    frame False {
                    }
                    frame True {
                      n401 = global read "Tick Count.vi" "Tick Count"() -> (w889:u64)
                      n402 = while {
                        shift-right: [w902] -> w888
                        shift-left: w890 -> [w894]
                        shift-right: [w897] -> _
                        shift-left: w889 -> [w896]
                        stop <- w891 stop-if-true
                        n403 = local read "External Pause"() -> (w901:bool)
                        n404 = local read "Internal Pause"() -> (w899:bool)
                        n405 = global read "Tick Count.vi" "Tick Count"() -> (w897:u64)
                        n406 = local read "External Stop"() -> (w893:bool)
                        n407 = Not(x=w901) -> (.not. x?=w900:bool)
                        n408 = Not(x=w899) -> (.not. x?=w898:bool)
                        n409 = Subtract(x=w897, y=w896) -> (x-y=w895:u64)
                        n410 = And(x=w900, y=w898) -> (x .and. y?=w892:bool)
                        n411 = Add(x=w895, y=w894) -> (x+y=w902:u64)
                        n412 = Or(x=w892, y=w893) -> (x .or. y?=w891:bool)
                      }
                    }
                  }
                }
                frame #1 {
                  n413 = global read "Tick Count.vi" "Tick Count"() -> (w907:u64)
                  n414 = Subtract(x=w907, y=w908) -> (x-y=w905:u64)
                  n415 = To Fixed-Point(number=w905) -> (fixed-point=w906:fxp<+,64,64>)  [unwired: 1 in]
                  n416 = case shown="True" "Change V on Fly" {
                    tunnel: w906 -> [w913 _]
                    tunnel: [w912 FALSE ("Finished Move")] -> w904
                    frame False {
                      n417 = local read "Jump V"() -> (w911:bool)
                      n418 = local read "V END"() -> (w910:i16)
                      n419 = case shown="True" w911 {
                        tunnel: w910 -> [w922 w923]
                        tunnel: [w921 w923] -> w909
                        tunnel: w913 -> [w920 _]
                        tunnel: [w919 TRUE ("Finished Move")] -> w912
                        frame False {
                          n420 = local read "ExpandVelScaller V"() -> (w914:i16)
                          n421 = local read "V VEl"() -> (w917:i16)
                          n422 = local read "V START"() -> (w918:i16)
                          n423 = Number To Boolean Array(number=w917) -> (Boolean array=w916:bool[])
                          n424 = Boolean Array To Number(Boolean array=w916) -> (number=w915:fxp<+/-,16,16>)
                          n425 = call "LinearMove.vi"("Time"=w920, "Start"=w918, "End"=w922, "Velocity"=w915, "ExpandVelScaller"=w914) -> ("OutPosition"=w921:i16, "Finished Move"=w919:bool)  [unwired: 13 in]
                        }
                        frame True {
                        }
                      }
                      n426 = local write "Applied Voltage"(w909) -> ()
                      n427 = xnode "FPGA I/O Node"("Connector0/AO3"=w909) -> ()  [unwired: 1 in, 1 out]
                    }
                    frame True {
                      n428 = local write "Applied Voltage"("V on Fly") -> ()
                      n429 = xnode "FPGA I/O Node"("Connector0/AO3"="V on Fly") -> ()  [unwired: 1 in, 1 out]
                    }
                  }
                }
                frame #2 {
                  n430 = local read "OnlyStopLineONCE V"() -> (w929:bool)
                  n431 = case shown="False" w929 {
                    tunnel: [w934 FALSE ("EndCurrentLine")] -> w930
                    frame False {
                      n432 = local read "EndCurrentLine"() -> (w934:bool)
                      n433 = case shown="True" w934 {
                        frame False {
                        }
                        frame True {
                          n434 = local write "OnlyStopLineONCE V"(TRUE ("EndCurrentLine")) -> ()
                        }
                      }
                    }
                    frame True {
                    }
                  }
                  n435 = local read "External Stop"() -> (w931:bool)
                  n436 = Or(x=w927, y=w930) -> (x .or. y?=w932:bool)
                  n437 = Or(x=w931, y=w932) -> (x .or. y?=w928:bool)
                }
              }
              n438 = local write "StopMoveV"(w876) -> ()
            }
          }
          frame True {
          }
        }
        n439 = case shown="False" w222 {
          tunnel: w217 -> [w822 _]
          frame False {
            n440 = while {
              shift-right: [w824] -> _
              shift-left: w822 -> [w827]
              stop <- w823 stop-if-true
              n441 = flat-sequence {
                tunnel: w827 -> [w829]
                tunnel: [w830] -> w828
                tunnel: w828 -> [w864]
                tunnel: [w864] -> w826
                tunnel: [w861] -> w825
                tunnel: [w871] -> w824
                tunnel: w826 -> [w871]
                tunnel: w825 -> [w865]
                tunnel: [w866] -> w823
                frame #0 {
                  n442 = local read "Internal Pause"() -> (w832:bool)
                  n443 = local read "External Pause"() -> (w833:bool)
                  n444 = Or(x=w833, y=w832) -> (x .or. y?=w831:bool)
                  n445 = case shown="True" w831 {
                    tunnel: w829 -> [w834 w837]
                    tunnel: [w834 w835] -> w830
                    frame False {
                    }
                    frame True {
                      n446 = global read "Tick Count.vi" "Tick Count"() -> (w836:u64)
                      n447 = while {
                        shift-right: [w849] -> w835
                        shift-left: w837 -> [w841]
                        shift-right: [w844] -> _
                        shift-left: w836 -> [w843]
                        stop <- w838 stop-if-true
                        n448 = local read "External Pause"() -> (w848:bool)
                        n449 = local read "Internal Pause"() -> (w846:bool)
                        n450 = global read "Tick Count.vi" "Tick Count"() -> (w844:u64)
                        n451 = local read "External Stop"() -> (w840:bool)
                        n452 = Not(x=w848) -> (.not. x?=w847:bool)
                        n453 = Not(x=w846) -> (.not. x?=w845:bool)
                        n454 = Subtract(x=w844, y=w843) -> (x-y=w842:u64)
                        n455 = And(x=w847, y=w845) -> (x .and. y?=w839:bool)
                        n456 = Add(x=w842, y=w841) -> (x+y=w849:u64)
                        n457 = Or(x=w839, y=w840) -> (x .or. y?=w838:bool)
                      }
                    }
                  }
                }
                frame #1 {
                  # "MAE 18/8/2014: Changed 0 to -32768 to allow -10 to 10V option. Note: as this is the full range of an I16 the coercion isn't doing much. In future make this boolean controlled from the T/F in advanced settings"
                  n458 = global read "Tick Count.vi" "Tick Count"() -> (w863:u64)
                  n459 = Subtract(x=w863, y=w864) -> (x-y=w850:u64)
                  n460 = To Fixed-Point(number=w850) -> (fixed-point=w862:fxp<+,64,64>)  [unwired: 1 in]
                  n461 = local read "X VEL"() -> (w854:i16)
                  n462 = local read "ExpandVelScaller X"() -> (w851:i16)
                  n463 = local read "X END"() -> (w852:i16)
                  n464 = local read "X START"() -> (w853:i16)
                  n465 = Number To Boolean Array(number=w854) -> (Boolean array=w860:bool[])
                  n466 = Boolean Array To Number(Boolean array=w860) -> (number=w859:fxp<+/-,16,16>)
                  n467 = call "LinearMove.vi"("Time"=w862, "Start"=w853, "End"=w852, "Velocity"=w859, "ExpandVelScaller"=w851) -> ("OutPosition"=w855:i16, "Finished Move"=w861:bool)  [unwired: 13 in]
                  n468 = In Range and Coerce(upper limit=i16 32767, x=w855, lower limit=i16 -32768) -> (coerced(x)=w856:i16)  [unwired: 1 out]
                  n469 = local write "Applied X"(w856) -> ()
                  n470 = xnode "I/O Node"("Connector0/AO0"=w856) -> ()  [unwired: 1 in, 1 out]
                }
                frame #2 {
                  n471 = local read "OnlyStopLineONCE X"() -> (w868:bool)
                  n472 = case shown="False" w868 {
                    tunnel: [w872 FALSE ("EndCurrentLine")] -> w867
                    frame False {
                      n473 = local read "EndCurrentLine"() -> (w872:bool)
                      n474 = case shown="True" w872 {
                        frame False {
                        }
                        frame True {
                          n475 = local write "OnlyStopLineONCE X"(TRUE ("EndCurrentLine")) -> ()
                        }
                      }
                    }
                    frame True {
                    }
                  }
                  n476 = local read "External Stop"() -> (w870:bool)
                  n477 = Or(x=w865, y=w867) -> (x .or. y?=w869:bool)
                  n478 = Or(x=w870, y=w869) -> (x .or. y?=w866:bool)
                }
              }
              n479 = local write "StopMoveX"(w823) -> ()
            }
          }
          frame True {
          }
        }
        n480 = case shown="False" w221 {
          tunnel: w217 -> [w769 _]
          frame False {
            n481 = while {
              shift-right: [w771] -> _
              shift-left: w769 -> [w774]
              stop <- w770 stop-if-true
              n482 = flat-sequence {
                tunnel: w774 -> [w776]
                tunnel: [w777] -> w775
                tunnel: w775 -> [w811]
                tunnel: [w811] -> w773
                tunnel: [w808] -> w772
                tunnel: [w818] -> w771
                tunnel: w773 -> [w818]
                tunnel: w772 -> [w812]
                tunnel: [w813] -> w770
                frame #0 {
                  n483 = local read "External Pause"() -> (w780:bool)
                  n484 = local read "Internal Pause"() -> (w779:bool)
                  n485 = Or(x=w780, y=w779) -> (x .or. y?=w778:bool)
                  n486 = case shown="True" w778 {
                    tunnel: w776 -> [w781 w784]
                    tunnel: [w781 w782] -> w777
                    frame False {
                    }
                    frame True {
                      n487 = global read "Tick Count.vi" "Tick Count"() -> (w783:u64)
                      n488 = while {
                        shift-right: [w796] -> w782
                        shift-left: w784 -> [w788]
                        shift-right: [w791] -> _
                        shift-left: w783 -> [w790]
                        stop <- w785 stop-if-true
                        n489 = local read "External Pause"() -> (w795:bool)
                        n490 = local read "Internal Pause"() -> (w793:bool)
                        n491 = global read "Tick Count.vi" "Tick Count"() -> (w791:u64)
                        n492 = local read "External Stop"() -> (w787:bool)
                        n493 = Not(x=w795) -> (.not. x?=w794:bool)
                        n494 = Not(x=w793) -> (.not. x?=w792:bool)
                        n495 = Subtract(x=w791, y=w790) -> (x-y=w789:u64)
                        n496 = And(x=w794, y=w792) -> (x .and. y?=w786:bool)
                        n497 = Add(x=w789, y=w788) -> (x+y=w796:u64)
                        n498 = Or(x=w786, y=w787) -> (x .or. y?=w785:bool)
                      }
                    }
                  }
                }
                frame #1 {
                  # "MAE 18/8/2014: Changed 0 to -32768 to allow -10 to 10V option. Note: as this is the full range of an I16 the coercion isn't doing much. In future make this boolean controlled from the T/F in advanced settings"
                  n499 = global read "Tick Count.vi" "Tick Count"() -> (w810:u64)
                  n500 = Subtract(x=w810, y=w811) -> (x-y=w797:u64)
                  n501 = To Fixed-Point(number=w797) -> (fixed-point=w809:fxp<+,64,64>)  [unwired: 1 in]
                  n502 = local read "Y VEL"() -> (w801:i16)
                  n503 = local read "ExpandVelScaller Y"() -> (w798:i16)
                  n504 = local read "Y END"() -> (w799:i16)
                  n505 = local read "Y START"() -> (w800:i16)
                  n506 = Number To Boolean Array(number=w801) -> (Boolean array=w807:bool[])
                  n507 = Boolean Array To Number(Boolean array=w807) -> (number=w806:fxp<+/-,16,16>)
                  n508 = call "LinearMove.vi"("Time"=w809, "Start"=w800, "End"=w799, "Velocity"=w806, "ExpandVelScaller"=w798) -> ("OutPosition"=w802:i16, "Finished Move"=w808:bool)  [unwired: 13 in]
                  n509 = In Range and Coerce(upper limit=i16 32767, x=w802, lower limit=i16 -32768) -> (coerced(x)=w803:i16)  [unwired: 1 out]
                  n510 = local write "Applied Y"(w803) -> ()
                  n511 = xnode "I/O Node"("Connector0/AO1"=w803) -> ()  [unwired: 1 in, 1 out]
                }
                frame #2 {
                  n512 = local read "OnlyStopLineONCE Y"() -> (w814:bool)
                  n513 = case shown="False" w814 {
                    tunnel: [w819 FALSE ("EndCurrentLine")] -> w815
                    frame False {
                      n514 = local read "EndCurrentLine"() -> (w819:bool)
                      n515 = case shown="True" w819 {
                        frame False {
                        }
                        frame True {
                          n516 = local write "OnlyStopLineONCE Y"(TRUE ("EndCurrentLine")) -> ()
                        }
                      }
                    }
                    frame True {
                    }
                  }
                  n517 = local read "External Stop"() -> (w817:bool)
                  n518 = Or(x=w812, y=w815) -> (x .or. y?=w816:bool)
                  n519 = Or(x=w817, y=w816) -> (x .or. y?=w813:bool)
                }
              }
              n520 = local write "StopMoveY"(w770) -> ()
            }
          }
          frame True {
          }
        }
        n521 = case shown="False" w220 {
          tunnel: w217 -> [w359 _]
          frame False {
            n522 = local read "Applied X"() -> (w358:i16)
            n523 = while {
              shift-right: [w363] -> _
              shift-left: w359 -> [w366]
              shift-right: [w360] -> _
              shift-left: w358 -> [w361]
              stop <- w362 stop-if-true
              n524 = flat-sequence {
                tunnel: w366 -> [w369]
                tunnel: [w370] -> w367
                tunnel: w367 -> [w407]
                tunnel: [w407] -> w365
                tunnel: [w402] -> w364
                tunnel: w361 -> [w396]
                tunnel: [w395] -> w360
                tunnel: [w765] -> w363
                tunnel: w365 -> [w765]
                tunnel: w364 -> [w759]
                tunnel: [w760] -> w362
                frame #0 {
                  n525 = local read "Update Position Loop Wait Time (ms)"() -> (w368:u16)
                  n526 = local read "External Pause"() -> (w373:bool)
                  n527 = local read "Internal Pause"() -> (w372:bool)
                  n528 = Or(x=w373, y=w372) -> (x .or. y?=w371:bool)
                  n529 = case shown="True" w371 {
                    tunnel: w369 -> [w374 w377]
                    tunnel: [w374 w375] -> w370
                    frame False {
                    }
                    frame True {
                      n530 = global read "Tick Count.vi" "Tick Count"() -> (w376:u64)
                      n531 = while {
                        shift-right: [w389] -> w375
                        shift-left: w377 -> [w381]
                        shift-right: [w384] -> _
                        shift-left: w376 -> [w383]
                        stop <- w378 stop-if-true
                        n532 = local read "External Pause"() -> (w388:bool)
                        n533 = local read "Internal Pause"() -> (w386:bool)
                        n534 = global read "Tick Count.vi" "Tick Count"() -> (w384:u64)
                        n535 = local read "External Stop"() -> (w380:bool)
                        n536 = Not(x=w388) -> (.not. x?=w387:bool)
                        n537 = Not(x=w386) -> (.not. x?=w385:bool)
                        n538 = Subtract(x=w384, y=w383) -> (x-y=w382:u64)
                        n539 = And(x=w387, y=w385) -> (x .and. y?=w379:bool)
                        n540 = Add(x=w382, y=w381) -> (x+y=w389:u64)
                        n541 = Or(x=w379, y=w380) -> (x .or. y?=w378:bool)
                      }
                    }
                  }
                  n542 = call "Loop Timer"("Count(mSec)"=w368) -> ()  [unwired: 1 out]
                }
                frame #1 {
                  # "MAE 18/8/2014: Changed 0 to -32768 to allow -10 to 10V option. Note: as this is the full range of an I16 the coercion isn't doing much. In future make this boolean controlled from the T/F in advanced settings"
                  n543 = global read "Tick Count.vi" "Tick Count"() -> (w406:u64)
                  n544 = local read "Feedback2 Boolean"() -> (w390:bool)
                  n545 = local read "LineType"() -> (w393:i16)
                  n546 = local read "Feedback1 Boolean"() -> (w391:bool)
                  n547 = Subtract(x=w406, y=w407) -> (x-y=w398:u64)
                  n548 = To Fixed-Point(number=w398) -> (fixed-point=w394:fxp<+,64,64>)  [unwired: 1 in]
                  n549 = Or(x=w391, y=w390) -> (x .or. y?=w392:bool)
                  n550 = case shown="15" w393 {
                    tunnel: "P" -> [_ _ _ w443 w455 w471 w492 _ w527 _ _ _ _]
                    tunnel: [w410 w420 w427 w438 w451 w466 w482 w515 w522 w544 w609 w682 w745] -> w402
                    tunnel: [w409 w419 w429 w441 w453 w469 w481 w518 w525 w546 w611 w684 w750] -> w401
                    tunnel: "Upper limit Of dZ" -> [_ _ _ w437 w452 w468 w491 _ w521 _ _ _ _]
                    tunnel: w396 -> [_ _ _ _ _ _ w489 _ _ _ _ _ _]
                    tunnel: [_ _ _ _ _ _ w488 _ _ _ _ _ _] -> w395
                    tunnel: w394 -> [w408 w418 w428 _ _ _ _ _ _ w545 w610 w683 _]
                    tunnel: w392 -> [_ w417 w427 _ _ _ _ _ _ _ _ _ _]
                    tunnel: w390 -> [_ _ _ _ _ _ _ _ w520 _ _ _ _]
                    frame 0, Default {
                      # "Normal Move"
                      n551 = local read "Z VEL"() -> (w413:i16)
                      n552 = local read "ExpandVelScaller Z"() -> (w416:i16)
                      n553 = local read "Z END"() -> (w415:i16)
                      n554 = local read "Z START"() -> (w414:i16)
                      n555 = Number To Boolean Array(number=w413) -> (Boolean array=w411:bool[])
                      n556 = Boolean Array To Number(Boolean array=w411) -> (number=w412:fxp<+/-,16,16>)
                      n557 = call "LinearMove.vi"("Time"=w408, "Start"=w414, "End"=w415, "Velocity"=w412, "ExpandVelScaller"=w416) -> ("OutPosition"=w409:i16, "Finished Move"=w410:bool)  [unwired: 13 in]
                    }
                    frame 1 {
                      # "Pause on Set Point"
                      n558 = local write "Internal Pause"(w417) -> ()
                      n559 = local read "Z VEL"() -> (w423:i16)
                      n560 = local read "ExpandVelScaller Z"() -> (w426:i16)
                      n561 = local read "Z END"() -> (w425:i16)
                      n562 = local read "Z START"() -> (w424:i16)
                      n563 = Number To Boolean Array(number=w423) -> (Boolean array=w421:bool[])
                      n564 = Boolean Array To Number(Boolean array=w421) -> (number=w422:fxp<+/-,16,16>)
                      n565 = call "LinearMove.vi"("Time"=w418, "Start"=w424, "End"=w425, "Velocity"=w422, "ExpandVelScaller"=w426) -> ("OutPosition"=w419:i16, "Finished Move"=w420:bool)  [unwired: 13 in]
                    }
                    frame 2 {
                      # "STOP Current Move on SetPoint"
                      n566 = local read "Z VEL"() -> (w432:i16)
                      n567 = local read "ExpandVelScaller Z"() -> (w435:i16)
                      n568 = local read "Z END"() -> (w434:i16)
                      n569 = local read "Z START"() -> (w433:i16)
                      n570 = Number To Boolean Array(number=w432) -> (Boolean array=w430:bool[])
                      n571 = Boolean Array To Number(Boolean array=w430) -> (number=w431:fxp<+/-,16,16>)
                      n572 = call "LinearMove.vi"("Time"=w428, "Start"=w433, "End"=w434, "Velocity"=w431, "ExpandVelScaller"=w435) -> ("OutPosition"=w429:i16)  [unwired: 13 in, 1 out]
                    }
                    frame 4 {
                      # "For scanning-Propotional Controller for constant distance scanning"
                      n573 = local read "Feedback1 Error"() -> (w436:i32)
                      n574 = Multiply(x=w443, y=w436) -> (x*y=w448:fxp<+/-,64,33>)
                      n575 = To Word Integer(number=w448) -> (16bit integer=w447:i16)
                      n576 = To Long Integer(number=w447) -> (32bit integer=w449:i32)
                      n577 = local read "StopMoveY"() -> (w439:bool)
                      n578 = local read "StopMoveX"() -> (w440:bool)
                      n579 = local read "Applied Z"() -> (w442:i16)
                      n580 = Negate(x=w437) -> (-x=w444:i32)
                      n581 = And(x=w440, y=w439) -> (x .and. y?=w438:bool)
                      n582 = In Range and Coerce(upper limit=w437, x=w449, lower limit=w444) -> (coerced(x)=w445:i32)  [unwired: 1 out]
                      n583 = To Long Integer(number=w442) -> (32bit integer=w446:i32)
                      n584 = Add(x=w446, y=w445) -> (x+y=w441:i32)
                    }
                    frame 11 {
                      # "Dependent on hold time-Propotional Controller for constant distance scanning"
                      n585 = local read "Feedback1 Error"() -> (w450:i32)
                      n586 = Multiply(x=w455, y=w450) -> (x*y=w460:fxp<+/-,64,33>)
                      n587 = To Word Integer(number=w460) -> (16bit integer=w459:i16)
                      n588 = To Long Integer(number=w459) -> (32bit integer=w461:i32)
                      n589 = local read "HasHeldHoldTimeHappend?"() -> (w451:bool)
                      n590 = local read "Applied Z"() -> (w454:i16)
                      n591 = Negate(x=w452) -> (-x=w456:i32)
                      n592 = In Range and Coerce(upper limit=w452, x=w461, lower limit=w456) -> (coerced(x)=w457:i32)  [unwired: 1 out]
                      n593 = To Long Integer(number=w454) -> (32bit integer=w458:i32)
                      n594 = Add(x=w458, y=w457) -> (x+y=w453:i32)
                    }
                    frame 10 {
                      # "deciding the limit of the Z movement (up or down) regardless of the x value"
                      # "convert the difference in siganls to distance in um"
                      # "External signal-Feedback_Threshold"
                      # "Dependent on holdtime-Propotional Controller for constant distance scanning ONLY for POSITIVE"
                      n595 = local read "Feedback1 Error"() -> (w462:i32)
                      n596 = Multiply(x=w471, y=w462) -> (x*y=w475:fxp<+/-,64,33>)
                      n597 = To Word Integer(number=w475) -> (16bit integer=w474:i16)
                      n598 = To Long Integer(number=w474) -> (32bit integer=w476:i32)
                      n599 = Negate(x=w468) -> (-x=w472:i32)
                      n600 = In Range and Coerce(upper limit=w468, x=w476, lower limit=w472) -> (coerced(x)=w464:i32)  [unwired: 1 out]
                      n601 = Less?(x=w464, y=0) -> (x < y?=w465:bool)
                      n602 = local read "HasHeldHoldTimeHappend?"() -> (w466:bool)
                      n603 = case shown="True" w465 {
                        tunnel: w464 -> [_ w478]
                        tunnel: [0 w478] -> w467
                        frame False {
                        }
                        frame True {
                        }
                      }
                      n604 = local read "Applied Z"() -> (w470:i16)
                      n605 = To Long Integer(number=w470) -> (32bit integer=w473:i32)
                      n606 = Add(x=w473, y=w467) -> (x+y=w469:i32)
                    }
                    frame 5 {
                      # "Proportional controller for constant distance scanning - with storing the positions in a buffer"
                      n607 = local read "Feedback1 Error"() -> (w479:i32)
                      n608 = local read "TraceRetraceFirstUse"() -> (w480:bool)
                      n609 = local read "Applied X"() -> (w488:i16)
                      n610 = local read "Applied Z"() -> (w490:i16)
                      n611 = Multiply(x=w492, y=w479) -> (x*y=w494:fxp<+/-,64,33>)
                      n612 = To Word Integer(number=w494) -> (16bit integer=w495:i16)
                      n613 = Subtract(x=w488, y=w489) -> (x-y=w487:i16)
                      n614 = To Long Integer(number=w495) -> (32bit integer=w493:i32)
                      n615 = case shown="False" w480 {
                        tunnel: w487 -> [w507 w510]
                        tunnel: [w506 w510] -> w486
                        tunnel: [w505 w509] -> w485
                        tunnel: w489 -> [w505 w508]
                        frame False {
                          n616 = Increment(x=w507) -> (x+1=w506:i16)
                        }
                        frame True {
                          n617 = Increment(x=w508) -> (x+1=w509:i16)
                        }
                      }
                      n618 = Negate(x=w491) -> (-x=w498:i32)
                      n619 = In Range and Coerce(upper limit=w491, x=w493, lower limit=w498) -> (coerced(x)=w497:i32)  [unwired: 1 out]
                      n620 = To Long Integer(number=w490) -> (32bit integer=w496:i32)
                      n621 = Add(x=w496, y=w497) -> (x+y=w481:i32)
                      n622 = for {
                        N: w486 -> [_]
                        shift-right: [w500] -> _
                        shift-left: w485 -> [w501]
                        tunnel: w481 -> [w504]
                        n623 = To Unsigned Long Integer(number=w501) -> (unsigned 32bit integer=w502:u32)
                        n624 = To Word Integer(number=w504) -> (16bit integer=w503:i16)
                        n625 = local write "TraceRetraceFirstUse"(TRUE ("TraceRetraceFirst?")) -> ()
                        n626 = xnode ("Memory Write")("Address"=w502, "Data"=w503) -> ()  [unwired: 1 in, 1 out]
                        n627 = Increment(x=w501) -> (x+1=w500:i16)
                      }
                      n628 = local read "StopMoveY"() -> (w483:bool)
                      n629 = local read "StopMoveX"() -> (w484:bool)
                      n630 = And(x=w484, y=w483) -> (x .and. y?=w482:bool)
                    }
                    frame 6 {
                      # "retrace the Z positions stored in the buffer, see feedbaack type 5"
                      n631 = local read "Applied X"() -> (w511:i16)
                      n632 = To Unsigned Long Integer(number=w511) -> (unsigned 32bit integer=w514:u32)
                      n633 = Add(x="Xoffset", y=w514) -> (x+y=w512:u32)
                      n634 = xnode ("Memory Read")("Address"=w512) -> ("Data"=w518:i16)  [unwired: 1 in, 1 out]
                      n635 = local read "StopMoveY"() -> (w516:bool)
                      n636 = local read "StopMoveX"() -> (w517:bool)
                      n637 = And(x=w517, y=w516) -> (x .and. y?=w515:bool)
                    }
                    frame 7 {
                      # "Proportianal controller for constant distance scan, with ability to pause based on a secondary signal"
                      n638 = local write "Internal Pause"(w520) -> ()
                      n639 = local read "Feedback1 Error"() -> (w519:i32)
                      n640 = Multiply(x=w527, y=w519) -> (x*y=w532:fxp<+/-,64,33>)
                      n641 = To Word Integer(number=w532) -> (16bit integer=w531:i16)
                      n642 = To Long Integer(number=w531) -> (32bit integer=w533:i32)
                      n643 = local read "StopMoveY"() -> (w523:bool)
                      n644 = local read "StopMoveX"() -> (w524:bool)
                      n645 = local read "Applied Z"() -> (w526:i16)
                      n646 = Negate(x=w521) -> (-x=w528:i32)
                      n647 = And(x=w524, y=w523) -> (x .and. y?=w522:bool)
                      n648 = In Range and Coerce(upper limit=w521, x=w533, lower limit=w528) -> (coerced(x)=w529:i32)  [unwired: 1 out]
                      n649 = To Long Integer(number=w526) -> (32bit integer=w530:i32)
                      n650 = Add(x=w530, y=w529) -> (x+y=w525:i32)
                    }
                    frame 8 {
                      # "Sum of most recent 1024"
                      n651 = local read "FeedBackType"() -> (w536:u8)
                      n652 = local read "Count Average"() -> (w537:i16)
                      n653 = case shown="1" w536 {
                        tunnel: [w549 w550 w551 w552 w553 w554] -> w535
                        frame 0, Default {
                          n654 = local read "Ext amp"() -> (w549:i16)
                        }
                        frame 1 {
                          n655 = local read "MeasuredCurrent"() -> (w550:i16)
                        }
                        frame 2 {
                          n656 = local read "MeasuredCurrent 2"() -> (w551:i16)
                        }
                        frame 3 {
                          n657 = local read "Ext Phase"() -> (w552:i16)
                        }
                        frame 4 {
                          n658 = local read "MeasuredCurrent"() -> (w553:i16)
                        }
                        frame 5 {
                          n659 = local read "MeasuredCurrent 2"() -> (w554:i16)
                        }
                      }
                      n660 = Equal?(x=w537, y="P2AvgWhole") -> (x = y?=w547:bool)
                      n661 = local read "ExtraTime 2"() -> (w540:fxp<+,64,64>)
                      n662 = To Long Integer(number=w535) -> (32bit integer=w534:i32)
                      n663 = local read "AverageSum"() -> (w543:i64)
                      n664 = case shown="True" w547 {
                        tunnel: w534 -> [w563 w584]
                        tunnel: w543 -> [w564 w591]
                        tunnel: [w565 w591] -> w548
                        tunnel: w537 -> [w562 w578]
                        tunnel: [w561 w578] -> w542
                        tunnel: [w560 w592] -> w546
                        tunnel: w545 -> [w558 w586]
                        tunnel: [FALSE w580] -> w544
                        tunnel: [w558 w588] -> w541
                        tunnel: w540 -> [_ w588]
                        tunnel: [w555 w576] -> w539
                        frame False {
                          n665 = local read "SampleIterator"() -> (w555:i16)
                          n666 = local read "IterateHolder"() -> (w557:i16)
                          n667 = Less?(x=w555, y=w557) -> (x < y?=w556:bool)
                          n668 = case shown="True" w556 {
                            tunnel: [w566 w573] -> w565
                            tunnel: w564 -> [w566 w572]
                            tunnel: w563 -> [_ w568]
                            tunnel: w562 -> [w567 w570]
                            tunnel: [w567 w571] -> w561
                            frame False {
                            }
                            frame True {
                              # "Count up to 1024 (start at 0) data points then start moving"
                              n669 = To Quad Integer(1:w568) -> (0:w569:i64)
                              n670 = Increment(x=w570) -> (x+1=w571:i16)
                              n671 = Add(x=w572, y=w569) -> (x+y=w573:i64)
                            }
                          }
                          n672 = local read "Applied Z"() -> (w560:i16)
                        }
                        frame True {
                          # "STOP Current Move on SetPoint"
                          n673 = local read "AverageSum"() -> (w590:i64)
                          n674 = local read "Feedback_Threshold"() -> (w575:i64)
                          n675 = Subtract(x=w586, y=w588) -> (x-y=w589:fxp<+/-,64,65>)
                          n676 = Scale By Power Of 2(n="P2AvgMinus", x=w590) -> (x*2^n=w579:i64)
                          n677 = To Fixed-Point(fixed-point type=w586, number=w589) -> (fixed-point=w587:fxp<+,64,64>)
                          n678 = To Long Integer(number=w575) -> (32bit integer=w574:i32)
                          n679 = local read "Z VEL"() -> (w595:i16)
                          n680 = Subtract(x=w579, y=w574) -> (x-y=w585:i64)
                          n681 = local read "ExpandVelScaller Z"() -> (w598:i16)
                          n682 = local read "Z END"() -> (w597:i16)
                          n683 = local read "Z START"() -> (w596:i16)
                          n684 = Number To Boolean Array(number=w595) -> (Boolean array=w593:bool[])
                          n685 = Add(x=w574, y=w579) -> (x+y=w583:i64)
                          n686 = Boolean Array To Number(Boolean array=w593) -> (number=w594:fxp<+/-,16,16>)
                          n687 = Greater?(x=w584, y=w583) -> (0:w582:bool)
                          n688 = call "LinearMove.vi"("Time"=w587, "Start"=w596, "End"=w597, "Velocity"=w594, "ExpandVelScaller"=w598) -> ("OutPosition"=w592:i16)  [unwired: 13 in, 1 out]
                          n689 = Less?(x=w584, y=w585) -> (x < y?=w581:bool)
                          n690 = Or(x=w582, y=w581) -> (x .or. y?=w580:bool)
                          n691 = local read "SampleNum"() -> (w576:i16)
                        }
                      }
                      "ExtraTime 2" <- w541
                      n692 = local write "IterateHolder"(w539) -> ()
                      n693 = local write "AverageSum"(w548) -> ()
                      n694 = local write "Count Average"(w542) -> ()
                    }
                    frame 9 {
                      # "Sum of most recent 1024"
                      n695 = local read "FeedBackType"() -> (w601:u8)
                      n696 = local read "P2AvgWhole"() -> (w602:i32)
                      n697 = local read "Count Average"() -> (w606:i16)
                      n698 = case shown="1" w601 {
                        tunnel: [w614 w615 w616 w617 w618 w619] -> w600
                        frame 0, Default {
                          n699 = local read "Ext amp"() -> (w614:i16)
                        }
                        frame 1 {
                          n700 = local read "MeasuredCurrent"() -> (w615:i16)
                        }
                        frame 2 {
                          n701 = local read "MeasuredCurrent 2"() -> (w616:i16)
                        }
                        frame 3 {
                          n702 = local read "Ext Phase"() -> (w617:i16)
                        }
                        frame 4 {
                          n703 = local read "MeasuredCurrent"() -> (w618:i16)
                        }
                        frame 5 {
                          n704 = local read "MeasuredCurrent 2"() -> (w619:i16)
                        }
                      }
                      n705 = Equal?(x=w606, y=w602) -> (x = y?=w612:bool)
                      n706 = local read "ExtraTime 3"() -> (w604:fxp<+,64,64>)
                      n707 = To Long Integer(number=w600) -> (32bit integer=w599:i32)
                      n708 = local read "AverageSum"() -> (w608:i64)
                      n709 = case shown="True" w612 {
                        tunnel: w599 -> [w628 w641]
                        tunnel: w608 -> [w629 _]
                        tunnel: [w630 w643] -> w613
                        tunnel: w606 -> [w627 w649]
                        tunnel: [w626 w649] -> w607
                        tunnel: [w625 w659] -> w611
                        tunnel: w610 -> [w623 w655]
                        tunnel: [FALSE w650] -> w609
                        tunnel: [w623 w657] -> w605
                        tunnel: w604 -> [_ w657]
                        tunnel: [w620 w646] -> w603
                        frame False {
                          n710 = local read "SampleIterator"() -> (w620:i16)
                          n711 = local read "IterateHolder"() -> (w622:i16)
                          n712 = Less?(x=w620, y=w622) -> (x < y?=w621:bool)
                          n713 = case shown="True" w621 {
                            tunnel: [w631 w638] -> w630
                            tunnel: w629 -> [w631 w637]
                            tunnel: w628 -> [_ w636]
                            tunnel: w627 -> [w632 w634]
                            tunnel: [w632 w633] -> w626
                            frame False {
                            }
                            frame True {
                              # "Count up to 1024 (start at 0) data points then start moving"
                              n714 = To Quad Integer(1:w636) -> (0:w635:i64)
                              n715 = Increment(x=w634) -> (x+1=w633:i16)
                              n716 = Add(x=w637, y=w635) -> (x+y=w638:i64)
                            }
                          }
                          n717 = local read "Applied Z"() -> (w625:i16)
                        }
                        frame True {
                          # "STOP Current Move on SetPoint"
                          n718 = local read "AverageSum"() -> (w645:i64)
                          n719 = local read "P2AvgMinus"() -> (w642:i32)
                          n720 = local read "Feedback_Threshold"() -> (w640:i64)
                          n721 = To Long Integer(number=w640) -> (32bit integer=w639:i32)
                          n722 = Subtract(x=w655, y=w657) -> (x-y=w658:fxp<+/-,64,65>)
                          n723 = Scale By Power Of 2(n=w642, x=w645) -> (x*2^n=w644:i64)
                          n724 = Subtract(x=w644, y=w639) -> (x-y=w654:i64)
                          n725 = local read "SampleIterator"() -> (w646:i16)
                          n726 = To Fixed-Point(fixed-point type=w655, number=w658) -> (fixed-point=w656:fxp<+,64,64>)
                          n727 = local read "IterateHolder"() -> (w648:i16)
                          n728 = Add(x=w639, y=w644) -> (x+y=w653:i64)
                          n729 = local read "Z VEL"() -> (w662:i16)
                          n730 = Less?(x=w646, y=w648) -> (x < y?=w647:bool)
                          "x < y?" <- w647
                          n731 = Greater?(x=w641, y=w653) -> (0:w652:bool)
                          n732 = local read "ExpandVelScaller Z"() -> (w665:i16)
                          n733 = local read "Z END"() -> (w664:i16)
                          n734 = Less?(x=w641, y=w654) -> (x < y?=w651:bool)
                          n735 = local read "Z START"() -> (w663:i16)
                          n736 = Or(x=w652, y=w651) -> (x .or. y?=w650:bool)
                          n737 = Number To Boolean Array(number=w662) -> (Boolean array=w660:bool[])
                          n738 = Boolean Array To Number(Boolean array=w660) -> (number=w661:fxp<+/-,16,16>)
                          n739 = call "LinearMove.vi"("Time"=w656, "Start"=w663, "End"=w664, "Velocity"=w661, "ExpandVelScaller"=w665) -> ("OutPosition"=w659:i16)  [unwired: 13 in, 1 out]
                          n740 = case shown="True" w647 {
                            tunnel: w645 -> [w666 w671]
                            tunnel: w644 -> [_ w670]
                            tunnel: [w666 w668] -> w643
                            tunnel: w641 -> [_ w667]
                            frame False {
                            }
                            frame True {
                              n741 = Subtract(x=w671, y=w670) -> (x-y=w669:i64)
                              n742 = Add(x=w669, y=w667) -> (x+y=w668:i64)
                            }
                          }
                        }
                      }
                      "ExtraTime 3" <- w605
                      n743 = local write "IterateHolder"(w603) -> ()
                      n744 = local write "AverageSum"(w613) -> ()
                      n745 = local write "Count Average"(w607) -> ()
                    }
                    frame 14 {
                      # "Sum of most recent 1024"
                      n746 = local read "FeedBackType"() -> (w674:u8)
                      n747 = local read "Count Average"() -> (w676:i16)
                      n748 = local read "P2AvgWhole"() -> (w675:i32)
                      n749 = case shown="1" w674 {
                        tunnel: [w687 w688 w689 w690 w691 w692] -> w673
                        frame 0, Default {
                          n750 = local read "Ext amp"() -> (w687:i16)
                        }
                        frame 1 {
                          n751 = local read "MeasuredCurrent"() -> (w688:i16)
                        }
                        frame 2 {
                          n752 = local read "MeasuredCurrent 2"() -> (w689:i16)
                        }
                        frame 3 {
                          n753 = local read "Ext Phase"() -> (w690:i16)
                        }
                        frame 4 {
                          n754 = local read "MeasuredCurrent"() -> (w691:i16)
                        }
                        frame 5 {
                          n755 = local read "MeasuredCurrent 2"() -> (w692:i16)
                        }
                      }
                      n756 = Equal?(x=w676, y=w675) -> (x = y?=w685:bool)
                      n757 = local read "ExtraTime 4"() -> (w678:fxp<+,64,64>)
                      n758 = To Long Integer(number=w673) -> (32bit integer=w672:i32)
                      n759 = local read "AverageSum"() -> (w681:i64)
                      n760 = case shown="True" w685 {
                        tunnel: w672 -> [w701 w730]
                        tunnel: w681 -> [w702 w736]
                        tunnel: [w703 w736] -> w686
                        tunnel: w676 -> [w700 w726]
                        tunnel: [w699 w726] -> w680
                        tunnel: [w698 w737] -> w684
                        tunnel: w683 -> [w696 w731]
                        tunnel: [FALSE w727] -> w682
                        tunnel: [w696 w733] -> w679
                        tunnel: w678 -> [_ w733]
                        tunnel: [w693 w725] -> w677
                        frame False {
                          n761 = local read "SampleIterator"() -> (w693:i16)
                          n762 = local read "IterateHolder"() -> (w695:i16)
                          n763 = Less?(x=w693, y=w695) -> (x < y?=w694:bool)
                          n764 = case shown="True" w694 {
                            tunnel: [w704 w711] -> w703
                            tunnel: w702 -> [w704 w710]
                            tunnel: w701 -> [_ w706]
                            tunnel: w700 -> [w705 w708]
                            tunnel: [w705 w709] -> w699
                            frame False {
                            }
                            frame True {
                              # "Count up to 1024 (start at 0) data points then start moving"
                              n765 = To Quad Integer(1:w706) -> (0:w707:i64)
                              n766 = Increment(x=w708) -> (x+1=w709:i16)
                              n767 = Add(x=w710, y=w707) -> (x+y=w711:i64)
                            }
                          }
                          n768 = local read "Applied Z"() -> (w698:i16)
                        }
                        frame True {
                          # "STOP Current Move on SetPoint"
                          n769 = local read "P2AvgMinus"() -> (w713:i32)
                          n770 = local read "Feedback_Threshold"() -> (w712:i64)
                          n771 = local read "AverageSum"() -> (w735:i64)
                          n772 = Subtract(x=w731, y=w733) -> (x-y=w734:fxp<+/-,64,65>)
                          n773 = To Quad Integer(1:w730) -> (0:w724:i64)
                          n774 = Scale By Power Of 2(n=w713, x=w735) -> (x*2^n=w720:i64)
                          n775 = To Fixed-Point(fixed-point type=w731, number=w734) -> (fixed-point=w732:fxp<+,64,64>)
                          n776 = To Quad Integer(1:w720) -> (0:w721:i64)
                          n777 = To Quad Integer(1:w712) -> (0:w716:i64)
                          n778 = Scale By Power Of 2(n=i16 15, x=w724) -> (x*2^n=w714:i64)
                          n779 = Scale By Power Of 2(n=i16 15, x=w721) -> (x*2^n=w715:i64)
                          n780 = local read "Z VEL"() -> (w740:i16)
                          n781 = local read "ExpandVelScaller Z"() -> (w743:i16)
                          n782 = Multiply(x=w720, y=w716) -> (x*y=w718:i64)
                          n783 = local read "Z END"() -> (w742:i16)
                          n784 = local read "Z START"() -> (w741:i16)
                          n785 = Number To Boolean Array(number=w740) -> (Boolean array=w738:bool[])
                          n786 = Add(x=w715, y=w718) -> (x+y=w719:i64)
                          n787 = Boolean Array To Number(Boolean array=w738) -> (number=w739:fxp<+/-,16,16>)
                          n788 = Subtract(x=w715, y=w718) -> (x-y=w717:i64)
                          n789 = Greater?(x=w714, y=w719) -> (0:w729:bool)
                          n790 = call "LinearMove.vi"("Time"=w732, "Start"=w741, "End"=w742, "Velocity"=w739, "ExpandVelScaller"=w743) -> ("OutPosition"=w737:i16)  [unwired: 13 in, 1 out]
                          n791 = Less?(x=w714, y=w717) -> (x < y?=w728:bool)
                          n792 = Or(x=w729, y=w728) -> (x .or. y?=w727:bool)
                          n793 = local read "SampleNum"() -> (w725:i16)
                        }
                      }
                      "ExtraTime 4" <- w679
                      n794 = local write "AverageSum"(w686) -> ()
                      n795 = local write "Count Average"(w680) -> ()
                      n796 = local write "IterateHolder"(w677) -> ()
                    }
                    frame 15 {
                      # "Charge accumulator\nKM 25/11/22"
                      n797 = local read "FeedBackType"() -> (w751:u8)
                      n798 = case shown="1" w751 {
                        tunnel: [w753 w754 w755 w756 w757 w758] -> w748
                        frame 0, Default {
                          n799 = local read "Ext amp"() -> (w753:i16)
                        }
                        frame 1 {
                          n800 = local read "MeasuredCurrent"() -> (w754:i16)
                        }
                        frame 2 {
                          n801 = local read "MeasuredCurrent 2"() -> (w755:i16)
                        }
                        frame 3 {
                          n802 = local read "Ext Phase"() -> (w756:i16)
                        }
                        frame 4 {
                          n803 = local read "MeasuredCurrent"() -> (w757:i16)
                        }
                        frame 5 {
                          n804 = local read "MeasuredCurrent 2"() -> (w758:i16)
                        }
                      }
                      n805 = local read "AverageSum"() -> (w752:i64)
                      n806 = local read "Feedback_Threshold 2"() -> (w744:i32)
                      n807 = To Quad Integer(1:w748) -> (0:w749:i64)
                      n808 = Add(x=w752, y=w749) -> (x+y=w747:i64)
                      n809 = local write "AverageSum"(w747) -> ()
                      n810 = Absolute Value(x=w747) -> (abs(x)=w746:i64)
                      n811 = Greater?(x=w746, y=w744) -> (0:w745:bool)
                      n812 = local read "Applied Z"() -> (w750:i16)
                    }
                  }
                  n813 = In Range and Coerce(upper limit=32767, x=w401, lower limit=-32768) -> (coerced(x)=w400:i32)  [unwired: 1 out]
                  n814 = To Word Integer(number=w400) -> (16bit integer=w399:i16)
                  n815 = xnode "I/O Node"("Connector0/AO2"=w399) -> ()  [unwired: 1 in, 1 out]
                  n816 = local write "Applied Z"(w399) -> ()
                }
                frame #2 {
                  n817 = local read "OnlyStopLineONCE Z"() -> (w762:bool)
                  n818 = case shown="True" w762 {
                    tunnel: [w766 FALSE ("EndCurrentLine")] -> w761
                    frame False {
                      n819 = local read "EndCurrentLine"() -> (w766:bool)
                      n820 = case shown="True" w766 {
                        frame False {
                        }
                        frame True {
                          n821 = local write "OnlyStopLineONCE Z"(TRUE ("EndCurrentLine")) -> ()
                        }
                      }
                    }
                    frame True {
                    }
                  }
                  n822 = local read "External Stop"() -> (w764:bool)
                  n823 = Or(x=w759, y=w761) -> (x .or. y?=w763:bool)
                  n824 = Or(x=w764, y=w763) -> (x .or. y?=w760:bool)
                }
              }
              n825 = local write "StopMoveZ"(w362) -> ()
            }
          }
          frame True {
          }
        }
        n826 = case shown="False" w219 {
          tunnel: w217 -> [w296 _]
          frame False {
            n827 = while {
              shift-right: [w298] -> _
              shift-left: w296 -> [w301]
              stop <- w297 stop-if-true
              n828 = flat-sequence {
                tunnel: w301 -> [w303]
                tunnel: [w304] -> w302
                tunnel: w302 -> [w329]
                tunnel: [w329] -> w300
                tunnel: [w325] -> w299
                tunnel: [w354] -> w298
                tunnel: w300 -> [w354]
                tunnel: w299 -> [w348]
                tunnel: [w349] -> w297
                frame #0 {
                  n829 = local read "Internal Pause"() -> (w306:bool)
                  n830 = local read "External Pause"() -> (w307:bool)
                  n831 = Or(x=w307, y=w306) -> (x .or. y?=w305:bool)
                  n832 = case shown="True" w305 {
                    tunnel: w303 -> [w308 w311]
                    tunnel: [w308 w309] -> w304
                    frame False {
                    }
                    frame True {
                      n833 = global read "Tick Count.vi" "Tick Count"() -> (w310:u64)
                      n834 = while {
                        shift-right: [w323] -> w309
                        shift-left: w311 -> [w315]
                        shift-right: [w318] -> _
                        shift-left: w310 -> [w317]
                        stop <- w312 stop-if-true
                        n835 = local read "External Pause"() -> (w322:bool)
                        n836 = local read "Internal Pause"() -> (w320:bool)
                        n837 = global read "Tick Count.vi" "Tick Count"() -> (w318:u64)
                        n838 = local read "External Stop"() -> (w314:bool)
                        n839 = Not(x=w322) -> (.not. x?=w321:bool)
                        n840 = Not(x=w320) -> (.not. x?=w319:bool)
                        n841 = Subtract(x=w318, y=w317) -> (x-y=w316:u64)
                        n842 = And(x=w321, y=w319) -> (x .and. y?=w313:bool)
                        n843 = Add(x=w316, y=w315) -> (x+y=w323:u64)
                        n844 = Or(x=w313, y=w314) -> (x .or. y?=w312:bool)
                      }
                    }
                  }
                }
                frame #1 {
                  n845 = global read "Tick Count.vi" "Tick Count"() -> (w328:u64)
                  n846 = Subtract(x=w328, y=w329) -> (x-y=w326:u64)
                  n847 = To Fixed-Point(number=w326) -> (fixed-point=w327:fxp<+,64,64>)  [unwired: 1 in]
                  n848 = case shown="True" "Change V on Fly 2" {
                    tunnel: w327 -> [w334 _]
                    tunnel: [w333 FALSE ("Finished Move")] -> w325
                    frame False {
                      n849 = local read "V2 END"() -> (w331:i16)
                      n850 = local read "Jump V2"() -> (w332:bool)
                      n851 = case shown="True" w332 {
                        tunnel: w331 -> [w343 w344]
                        tunnel: [w342 w344] -> w330
                        tunnel: w334 -> [w341 _]
                        tunnel: [w340 TRUE ("Finished Move")] -> w333
                        frame False {
                          n852 = local read "ExpandVelScaller V2"() -> (w335:i16)
                          n853 = local read "V2 VEl"() -> (w338:i16)
                          n854 = local read "V2 START"() -> (w339:i16)
                          n855 = Number To Boolean Array(number=w338) -> (Boolean array=w337:bool[])
                          n856 = Boolean Array To Number(Boolean array=w337) -> (number=w336:fxp<+/-,16,16>)
                          n857 = call "LinearMove.vi"("Time"=w341, "Start"=w339, "End"=w343, "Velocity"=w336, "ExpandVelScaller"=w335) -> ("OutPosition"=w342:i16, "Finished Move"=w340:bool)  [unwired: 13 in]
                        }
                        frame True {
                        }
                      }
                      n858 = local write "Applied Voltage 2"(w330) -> ()
                      n859 = xnode "FPGA I/O Node"("Connector0/AO4"=w330) -> ()  [unwired: 1 in, 1 out]
                    }
                    frame True {
                      n860 = local write "Applied Voltage 2"("V2 on Fly") -> ()
                      n861 = xnode "FPGA I/O Node"("Connector0/AO4"="V2 on Fly") -> ()  [unwired: 1 in, 1 out]
                    }
                  }
                }
                frame #2 {
                  n862 = local read "OnlyStopLineONCE V2"() -> (w350:bool)
                  n863 = case shown="False" w350 {
                    tunnel: [w355 FALSE ("EndCurrentLine")] -> w351
                    frame False {
                      n864 = local read "EndCurrentLine"() -> (w355:bool)
                      n865 = case shown="True" w355 {
                        frame False {
                        }
                        frame True {
                          n866 = local write "OnlyStopLineONCE V2"(TRUE ("EndCurrentLine")) -> ()
                        }
                      }
                    }
                    frame True {
                    }
                  }
                  n867 = Or(x=w348, y=w351) -> (x .or. y?=w353:bool)
                  n868 = local read "External Stop"() -> (w352:bool)
                  n869 = Or(x=w352, y=w353) -> (x .or. y?=w349:bool)
                }
              }
              n870 = local write "StopMoveV2"(w297) -> ()
            }
          }
          frame True {
          }
        }
      }
    }
  }
  n871 = node-c288(w2) -> ()
